vi "MAIN_All_In_One.vi"() -> ()   [LabVIEW 2019]
uses:
  States/Assessment_Modes.ctl
  States/Main_States.ctl
  States/Hand.ctl
  States/ROM_States.ctl
  <vilib>/myRIO/Common/Instrument Driver Framework/myRIO v1.0/Encoder/typedefs/Encoder Signal Mode.ctl
  Shared VIs/Messages/NewPatientNotifierArgs.ctl
  Shared VIs/ModelSpecific/ETHMikeModel.ctl
  Shared VIs/ModelSpecific/ReadOnlyGlobalActions.ctl
  <vilib>/myRIO/Instrument Drivers/Onboard IO/AI/typedefs/AI Reference.ctl
  <vilib>/myRIO/Common/Instrument Driver Framework/Utilities/typedefs/myRIO Generic Hardware Reference.ctl
  <vilib>/myRIO/Common/Instrument Driver Framework/Utilities/typedefs/Hardware Version Enum.ctl
  <vilib>/myRIO/Common/Instrument Driver Framework/Utilities/typedefs/myRIO v1.0 Reference.ctl
  <vilib>/myRIO/Common/Instrument Driver Framework/Utilities/typedefs/Generic FPGA Reference.ctl
  <vilib>/myRIO/Common/Instrument Driver Framework/myRIO v1.0/AI/typedefs/AI Channels List.ctl
  <vilib>/myRIO/Common/Instrument Driver Framework/myRIO v1.0/AI/typedefs/AI Channels Enum.ctl
  <vilib>/myRIO/Common/Instrument Driver Framework/Utilities/typedefs/Analog Scaling Constants List.ctl
  <vilib>/myRIO/Common/Instrument Driver Framework/Utilities/typedefs/Analog Scaling Constants.ctl
  <vilib>/userDefined/High Color/nirio_resource_hc.ctl
  <vilib>/myRIO/Instrument Drivers/Onboard IO/AO/typedefs/AO Reference.ctl
  <vilib>/myRIO/Common/Instrument Driver Framework/myRIO v1.0/AO/typedefs/AO Channels List.ctl
  <vilib>/myRIO/Common/Instrument Driver Framework/myRIO v1.0/AO/typedefs/AO Channels Enum.ctl
  <vilib>/Platform/TimedLoop/XDataNode/timing_clust.ctl
  <vilib>/Platform/TimedLoop/XDataNode/nitl_modes.ctl
  <vilib>/Platform/TimedLoop/XDataNode/wakeup.ctl
  Shared VIs/TypeDef_TDMS_States.ctl
  <vilib>/Analysis/3filter.llb/Filter Passband Type.ctl
  Shared VIs/Messages/UdpGlobalActions.ctl
  Shared VIs/ENPID/OutputRange.ctl
  Shared VIs/Messages/MsgHeader.ctl
  Shared VIs/Messages/PatientSelectMsg.ctl
  Shared VIs/Messages/CommandMsg.ctl
  Shared VIs/Messages/BackendInfoMsg.ctl
  <vilib>/myRIO/Common/Instrument Driver Framework/myRIO v1.0/AI/vis/myRIO v1.1 Open AI.vi
  <vilib>/myRIO/Common/Instrument Driver Framework/myRIO v1.0/AO/vis/myRIO v1.1 Open AO.vi
  <vilib>/myRIO/Common/Instrument Driver Framework/Utilities/vis/Validate Channels.vi
  <vilib>/myRIO/Common/Instrument Driver Framework/myRIO v1.0/AI/vis/myRIO v1.0 Reserve AI.vi
  <vilib>/myRIO/Common/Instrument Driver Framework/myRIO v1.0/AO/vis/myRIO v1.0 Reserve AO.vi
  <vilib>/myRIO/Common/Instrument Driver Framework/myRIO v1.0/AI/vis/myRIO v1.0 Close AI.vi
  <vilib>/myRIO/Common/Instrument Driver Framework/myRIO v1.0/AO/vis/myRIO v1.0 Close AO.vi
  <vilib>/myRIO/Common/Instrument Driver Framework/myRIO v1.0/Encoder/vis/myRIO v1.0 Close Encoder.vi
  <vilib>/myRIO/Common/Instrument Driver Framework/myRIO v1.0/AI/vis/myRIO v1.0 Build MUX Configuration AI.vi
  <vilib>/myRIO/Common/Instrument Driver Framework/myRIO v1.0/Resource Manager/vis/myRIO v1.0 Reserve Channel List.vi
  <vilib>/myRIO/Common/Instrument Driver Framework/myRIO v1.0/AO/vis/myRIO v1.0 Build MUX Configuration AO.vi
  <vilib>/myRIO/Common/Instrument Driver Framework/myRIO v1.0/AI/vis/myRIO v1.0 Unreserve AI.vi
  <vilib>/myRIO/Common/Instrument Driver Framework/myRIO v1.0/AO/vis/myRIO v1.0 Unreserve AO.vi
  <vilib>/myRIO/Common/Instrument Driver Framework/myRIO v1.0/Encoder/vis/myRIO v1.0 Unreserve Encoder.vi
  <vilib>/myRIO/Common/Instrument Driver Framework/myRIO v1.0/Resource Manager/vis/myRIO v1.0 Reserve Channel.vi
  <vilib>/myRIO/Common/Instrument Driver Framework/myRIO v1.0/Resource Manager/vis/myRIO v1.0 Unreserve Channel.vi
  <vilib>/myRIO/Common/Instrument Driver Framework/myRIO v1.0/Resource Manager/vis/myRIO v1.0 Unreserve Channel List.vi
  <vilib>/myRIO/Common/Instrument Driver Framework/myRIO v1.0/Encoder/vis/myRIO v1.0 Build MUX Configuration Encoder.vi
  <vilib>/myRIO/Common/Instrument Driver Framework/myRIO v1.0/Resource Manager/vis/myRIO v1.0 Build Mutex Name.vi
  <vilib>/myRIO/Common/Instrument Driver Framework/myRIO v1.0/Resource Manager/vis/myRIO v1.0 Create Configuration List.vi
  <vilib>/Utility/VariantDataType/GetNumericInfo.vi
  <vilib>/Utility/error.llb/Error Cluster From Error Code.vi
  <vilib>/myRIO/Common/Instrument Driver Framework/myRIO v1.0/myRIO v1.1 Open.vi
  <vilib>/myRIO/Common/Instrument Driver Framework/myRIO v1.0/AO/vis/myRIO v1.0 Get Scaling Constants AO.vi
  <vilib>/myRIO/Common/Instrument Driver Framework/Utilities/vis/IO Manager.vi
  <vilib>/myRIO/Common/Instrument Driver Framework/Utilities/vis/Configuration Manager.vi
  <vilib>/myRIO/Common/Instrument Driver Framework/myRIO v1.0/myRIO v1.0 Close.vi
  <vilib>/myRIO/Common/Instrument Driver Framework/myRIO v1.0/AO/vis/myRIO v1.0 Write AO.vi
  <vilib>/myRIO/Common/Instrument Driver Framework/myRIO v1.0/AI/vis/myRIO v1.0 Get Scaling Constants AI.vi
  <vilib>/myRIO/Common/Instrument Driver Framework/myRIO v1.0/AI/vis/myRIO v1.0 Read AI.vi
  <vilib>/myRIO/Common/Instrument Driver Framework/myRIO v1.0/Encoder/vis/myRIO v1.0 Read Encoder.vi
  <vilib>/functionblocks/Counter/Elapsed Timer/Elapsed Timer.vi
  <vilib>/myRIO/Common/Instrument Driver Framework/myRIO v1.0/Encoder/vis/myRIO v1.0 Enable Encoder.vi
  <vilib>/myRIO/Common/Instrument Driver Framework/myRIO v1.0/Encoder/vis/myRIO v1.0 Shutdown Encoder.vi
  <vilib>/myRIO/Common/Instrument Driver Framework/myRIO v1.0/Resource Manager/vis/myRIO v1.0 Configure IO.vi
  <vilib>/myRIO/Instrument Drivers/Onboard IO/AO/vis/myRIO AO Open.xnode
  <vilib>/myRIO/Instrument Drivers/Onboard IO/AI/vis/myRIO AI Open.xnode
  <vilib>/platform/TimedLoop/XDataNode/XDataNode.xnode
  <vilib>/functionblocks/FB Core/FB Core.xnode
  <vilib>/myRIO/Instrument Drivers/Onboard IO/AO/AO.lvlib
  <vilib>/myRIO/Instrument Drivers/Onboard IO/Encoder/Encoder.lvlib
  <vilib>/myRIO/Instrument Drivers/Onboard IO/AI/AI.lvlib
  <vilib>/Platform/TimedLoop/XDataNode/XDNodeRunTimeDep.lvlib
  <vilib>/functionblocks/NI_FunctionBlock Libraries.lvlib
  <vilib>/addons/control/pid/NI_PID_pid.lvlib
  <vilib>/Analysis/NI_AALBase.lvlib
  <vilib>/ptbypt/NI_PtbyPt.lvlib
panel:
  out "SkipSignal":bool
  out "Force_calib_value":dbl
  out "Velocity_calib_value":dbl
  out "LogFileOpen":bool
  out "Phase Trial Count":i16
  out "Error which lead\nto TCP close":errorcluster
  out "TCP Error":errorcluster
  out "UDP Error":errorcluster
  in  "stop":bool
  out "SelectedHand":T1
  out "Connected":bool
  out "Remote IP":u32 format="%x"
  out "StopRequested":bool
  in  "TCP Server Port":u16=6662
  in  "UDP Destination Port":u16=6661
  out "DateTime":string
  out "SubjectNr":string
  out "StopSignal":bool
  out "RestartSignal":bool
  out "StartSignal":bool
  out "FrontendStartedSignal":bool
  out "Flexion":bool
  out "AssessmentFinished":bool
  out "ROM State":T2=enum."Passive"
  out "LeftHand":bool
  out "Task State":T3=enum."Start"
  out "MovingToTarget":bool=TRUE
  out "ROM max":dbl
  out "ROM min":dbl
  out "Zero Position":dbl
  out "Largest USB Partition Path":path
  out "Velocity unfiltered [deg/s]":dbl
  out "Trial Nr":i16
  out "Starting position":dbl
  out "Target Array":dbl[](array[numeric])
  out "AssessmentMode":T4
  out "Current Setpoint [A]":dbl
  out "Finished late?":bool
  out "Position [deg]":dbl
  out "Velocity [deg/s]":dbl
  out "Current [A]":dbl
  out "Time (s)":dbl
  out "Voltage force":dbl
  out "Force":dbl
  out "Force filtered":dbl
  out "Target state?":bool
  out "Target Position [deg]":dbl
  # "Frontend Connection"
  # "Command Signals"
  # "Motor State"
  # "Patient Data"
  # "Assessment State"
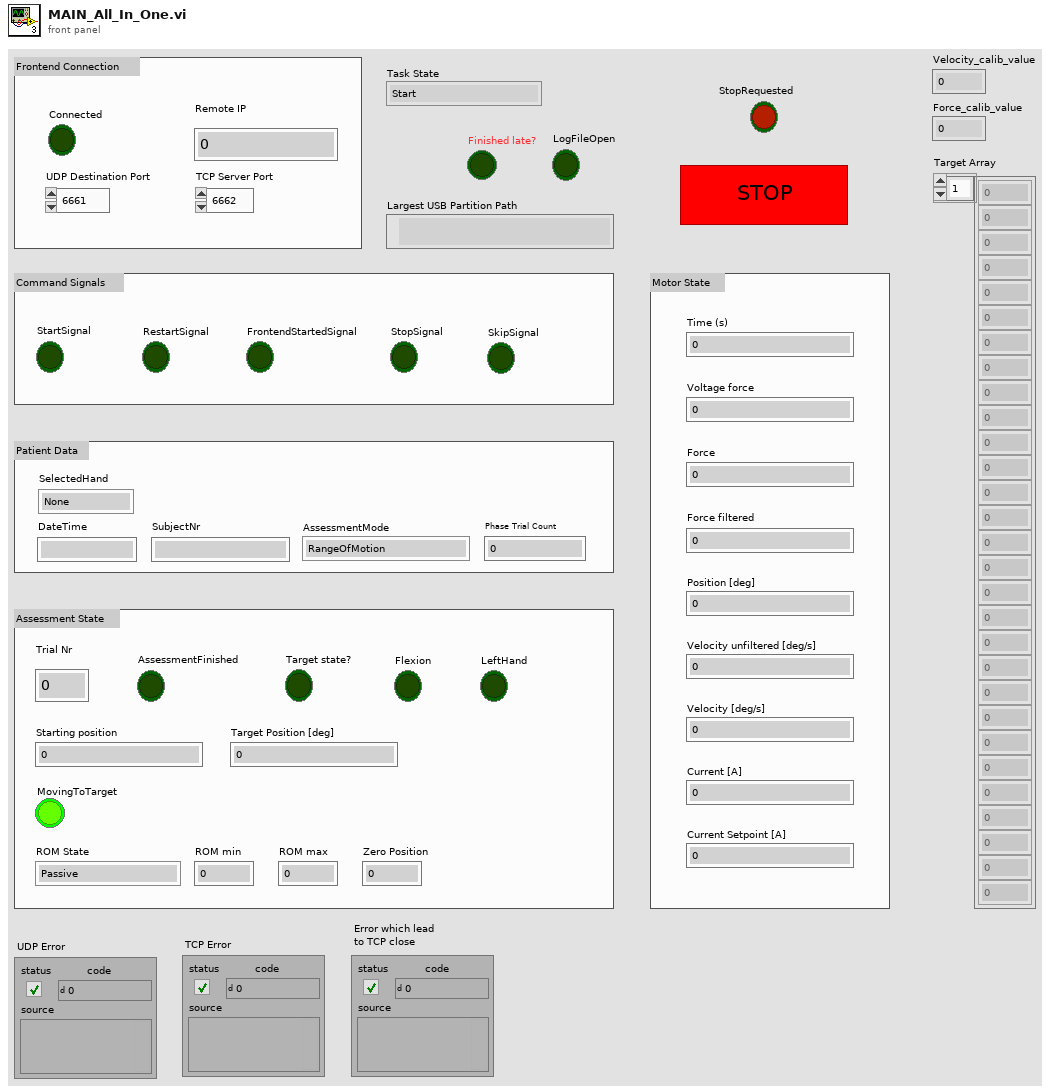
[diagram p1: front panel]
types:
  T1 = typedef "Hand.ctl" = enum8{"None", "Left", "Right"}
  T2 = typedef "ROM_States.ctl" = enum8{"Active", "Passive", "AutomaticPassive"}
  T3 = typedef "Main_States.ctl" = enum16{"Hand choice", "Start", "Show target", "Resetting", "WaitingForRestart"}
  T4 = typedef "Assessment_Modes.ctl" = enum8{"RangeOfMotion", "Force", "Motor", "Sensorimotor", "PositionMatching", "PreciseReaching"}
  T5 = typedef "NewPatientNotifierArgs.ctl" = cluster{"Left":bool, "Mode":T4, "Name":string, "Timestamp":string, "StudyName":string}
  T6 = cluster{"read mode":enum16{"polling", "blocking"}, "write mode":enum16{"polling", "blocking"}}
  T7 = typedef "nirio_resource_hc.ctl" = tag
  T8 = typedef "Hardware Version Enum.ctl" = enum16{"Unknown", "myRIO-1900", "myRIO-1950", "roboRIO", "NI ELVIS RIO CM", "ELVIS III"}
  T9 = typedef "TypeDef_TDMS_States.ctl" = enum16{"WaitingForCreate", "Create", "Buffering", "Flushing", "Write", "Close"}
  T10 = enum16{"open", "open or create", "create or replace", "create", "open (read-only)"}
  T11 = typedef "XDNodeRunTimeDep.lvlib/timing_clust.ctl" = cluster{"Expected End [f-1]":u64, "Actual End [f-1]":u64, "Finished Late? [f-1]":bool, "Expected End [i-1]":u64, "Actual End [i-1]":u64, "Finished Late? [i-1]":bool, "Expected Start [i]":u64, "Actual Start [i]":u64, "Expected Start [f]":u64, "Actual Start [f]":u64, "Source Name":string, "Structure Name":string, "Period":i64, "Deadline":i64, "Offset":i64, "Start":i64, "Priority":i32, "Timeout":i32, "Mode":T12, "Wakeup Reason":T13, "Error":errorcluster, "Source Type":string, "Secondary Source Type":string, "Global End Time":u64, "Global Start Time":u64, "Frame Duration":u64, "Iteration Duration":u64, "Assigned CPU":i32, "I/O Scan Engine Mode":u32}
  T12 = typedef "XDNodeRunTimeDep.lvlib/nitl_modes.ctl" = enum32{"No Change", "Process missed periods, maintain original phase", "Discard missed periods, maintain original phase", "Process missed periods, ignore original phase", "Discard missed periods, ignore original phase"}
  T13 = typedef "XDNodeRunTimeDep.lvlib/wakeup.ctl" = enum32{"Normal", "Aborted", "Asynchronous wakeup", "Timing source error", "Timed loop error", "Timeout"}
  T14 = enum8{"Invalid", "PatientSelect", "Command", "Skip", "BackendInfoReq", "UnknownOp (Must be Last)"}
  T15 = typedef "MsgHeader.ctl" = cluster{"MsgType [0]":u8, "MsgLen [1:2]":u16}
  T16 = typedef "PatientSelectMsg.ctl" = cluster{"LeftHand":bool, "AssessmentMode":u8, "SubjectNr":string, "DateTime":string, "PhaseTrialCount":i32, "StudyName":string}
  T17 = typedef "CommandMsg.ctl" = cluster{"EmergencyStop":bool, "Start":bool, "Restart":bool, "FrontendStarted":bool, "Close":bool}
  T18 = typedef "BackendInfoMsg.ctl" = cluster{"ProtocolVersion":u16, "DataPath":string}
  T19 = typedef "UdpGlobalActions.ctl" = enum16{"Read", "Write"}
  T20 = typedef "NI_AALBase.lvlib/Filter Passband Type.ctl" = enum32{"Lowpass", "Highpass", "Bandpass", "Bandstop"}
  T21 = typedef "ReadOnlyGlobalActions.ctl" = enum16{"Initialize", "Read"}
  T22 = typedef "ETHMikeModel.ctl" = enum16{"ETH Mike #1", "ETH Mike #2", "ETH Mike #3", "ETH Mike #4", "ETH MIKE #5"}
  T23 = typedef "Encoder Signal Mode.ctl" = enum16{"Quadrature phase signal", "Step and direction signal"}
  T24 = typedef "AO.lvlib/AO Reference.ctl" = cluster{"myRIO Reference":T25, "AO Channel List":T28, "AO Scaling Constant List":T30}
  T25 = typedef "myRIO Generic Hardware Reference.ctl" = cluster{"myRIO Model":T8, "myRIO Hardware Reference":T26}
  T26 = typedef "myRIO v1.0 Reference.ctl" = cluster{"Generic FPGA Reference":T27, "Allow multiple opens":bool}
  T27 = typedef "Generic FPGA Reference.ctl" = refnum<k20>
  T28 = typedef "AO Channels List.ctl" = T29[]
  T29 = typedef "AO Channels Enum.ctl" = enum16{"Not Connected", "AudioOut/Left", "AudioOut/Right", "C/AO0", "C/AO1", "A/AO0", "A/AO1", "B/AO0", "B/AO1"}
  T30 = typedef "Analog Scaling Constants List.ctl" = T31[]
  T31 = typedef "Analog Scaling Constants.ctl" = cluster{"LSB Weight (Volts)":dbl, "Offset (Volts)":dbl, "Signed?":bool}
  T32 = typedef "Encoder.lvlib/Encoder Reference.ctl" = cluster{"myRIO Reference":T25, "Encoder Channels Enum":T33}
  T33 = typedef "Encoder Channels Enum.ctl" = enum16{"Not Connected", "C/ENC0", "C/ENC1", "A/ENC", "A/ENC0", "A/ENC1", "A/ENC2", "A/ENC3", "A/ENC4", "A/ENC5", "A/ENC6", "A/ENC7", "A/ENC8", "A/ENC9", "B/ENC", "B/ENC0", "B/ENC1", "B/ENC2", "B/ENC3", "B/ENC4", "B/ENC5", "B/ENC6", "B/ENC7", "B/ENC8", "B/ENC9", "DIO/ENC0", "DIO/ENC1", "DIO/ENC2", "DIO/ENC3", "DIO/ENC4"}
  T34 = typedef "AI.lvlib/AI Reference.ctl" = cluster{"myRIO Reference":T25, "AI Channels List":T35, "AI Scaling Constants List":T30}
  T35 = typedef "AI Channels List.ctl" = T36[]
  T36 = typedef "AI Channels Enum.ctl" = enum16{"Not Connected", "AudioIn/Left", "AudioIn/Right", "C/AI0", "C/AI1", "A/AI0", "A/AI1", "A/AI2", "A/AI3", "A/AI4", "A/AI5", "A/AI6", "A/AI7", "B/AI0", "B/AI1", "B/AI2", "B/AI3", "B/AI4", "B/AI5", "B/AI6", "B/AI7", "AI/AI0", "AI/AI1", "AI/AI2", "AI/AI3", "A/AI0 (DIFF)", "A/AI1 (DIFF)", "A/AI2 (DIFF)", "A/AI3 (DIFF)", "B/AI0 (DIFF)", "B/AI1 (DIFF)", "B/AI2 (DIFF)", "B/AI3 (DIFF)"}
  T37 = typedef "LVAllMonitorsDisplayTypeDef.ctl" = cluster{"Bounds":cluster{"Left":i16, "Top":i16, "Right":i16, "Bottom":i16}, "Depth":i16}[]
  T38 = cluster{"Bounds":cluster{"Left":i16, "Top":i16, "Right":i16, "Bottom":i16}, "Depth":i16}
  T39 = cluster{"Left":i16, "Top":i16, "Right":i16, "Bottom":i16}
  T40 = enum16{"Standard", "Buffered", "CRLF", "Immediate"}
  T41 = typedef "UDPRobotState.ctl" = cluster{"Counter":u32, "Time":sgl, "Position":sgl, "StartingPosition":sgl, "TargetPosition":sgl, "Force":sgl, "TrialNr":u8, "RomState":u8, "TargetState":bool, "Finished":bool, "Flexion":bool}
  T42 = typedef "OutputRange.ctl" = cluster{"output high":dbl, "output low":dbl}
  T43 = typedef "Gains.ctl" = cluster{"K(e)":dbl, "Kp":dbl, "Ki":dbl, "Kd":dbl}
  T44 = typedef "NonLinearGainParams.ctl" = cluster{"Non-linear gain P":T45, "Non-linear gain I":T45, "Non-linear gain D":T45}
  T45 = typedef "NonLinearGain.ctl" = enum16{"exponential", "quadratic", "off"}
  T46 = typedef "DPartVariable.ctl" = enum16{"error", "process variable"}
  T47 = typedef "VelocityEstimate.ctl" = enum16{"derivative", "external"}
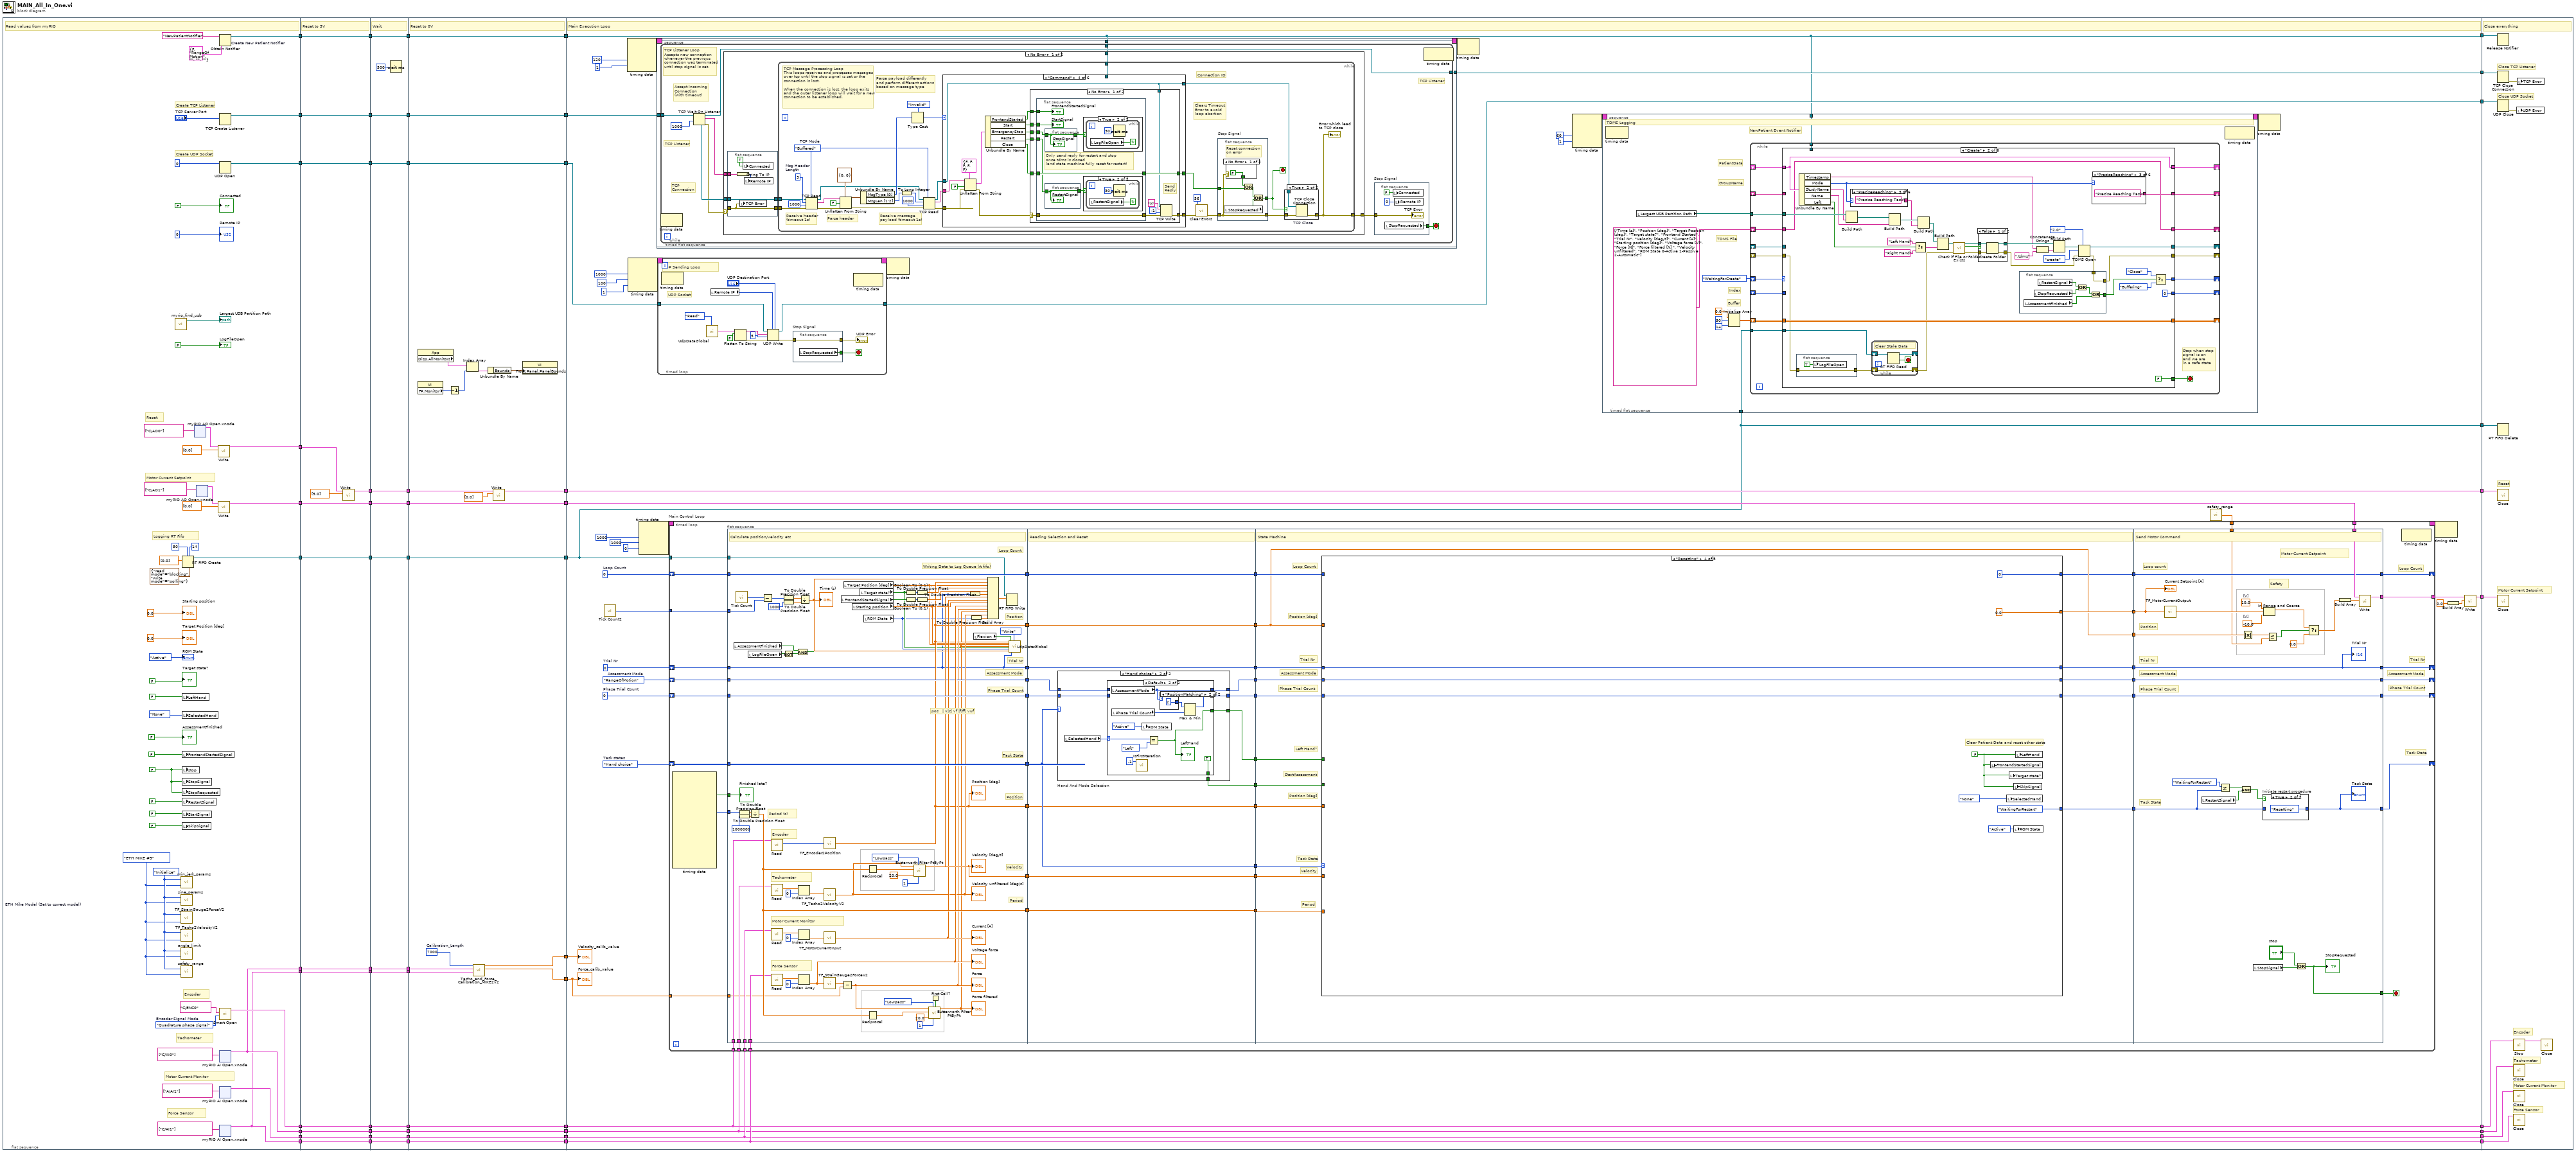
[diagram p0: block diagram]
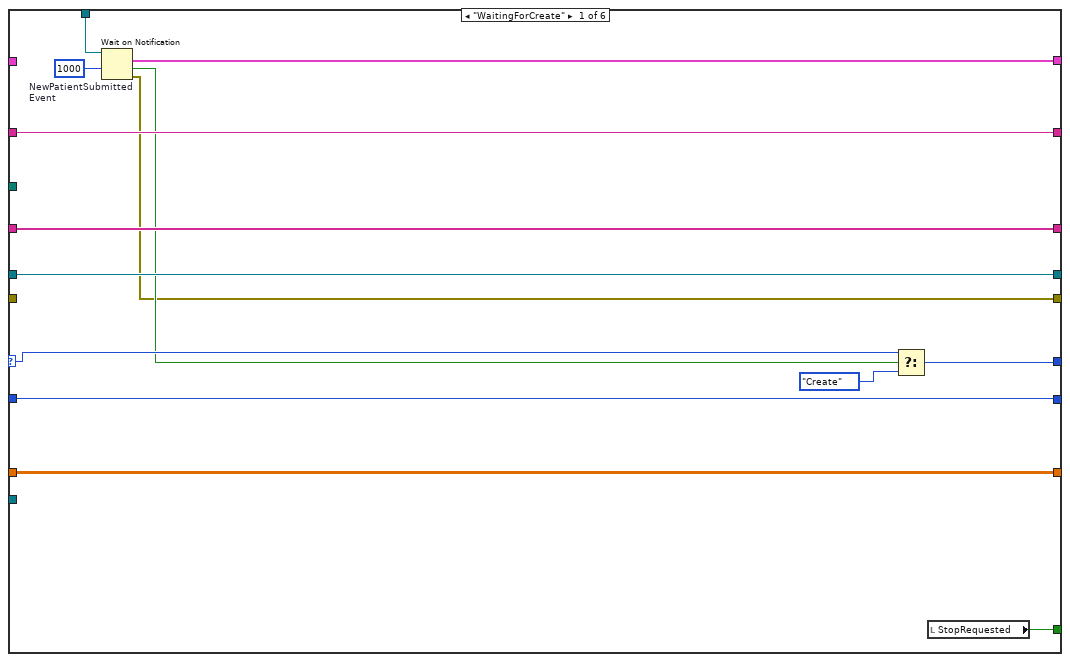
[diagram p2: hidden frame]
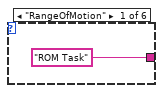
[diagram p3: hidden frame]
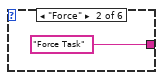
[diagram p4: hidden frame]
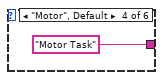
[diagram p5: hidden frame]
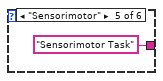
[diagram p6: hidden frame]
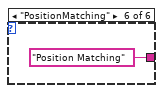
[diagram p7: hidden frame]
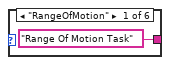
[diagram p9: hidden frame]
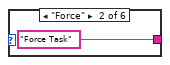
[diagram p10: hidden frame]
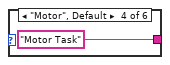
[diagram p11: hidden frame]
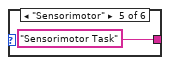
[diagram p12: hidden frame]
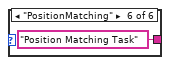
[diagram p13: hidden frame]
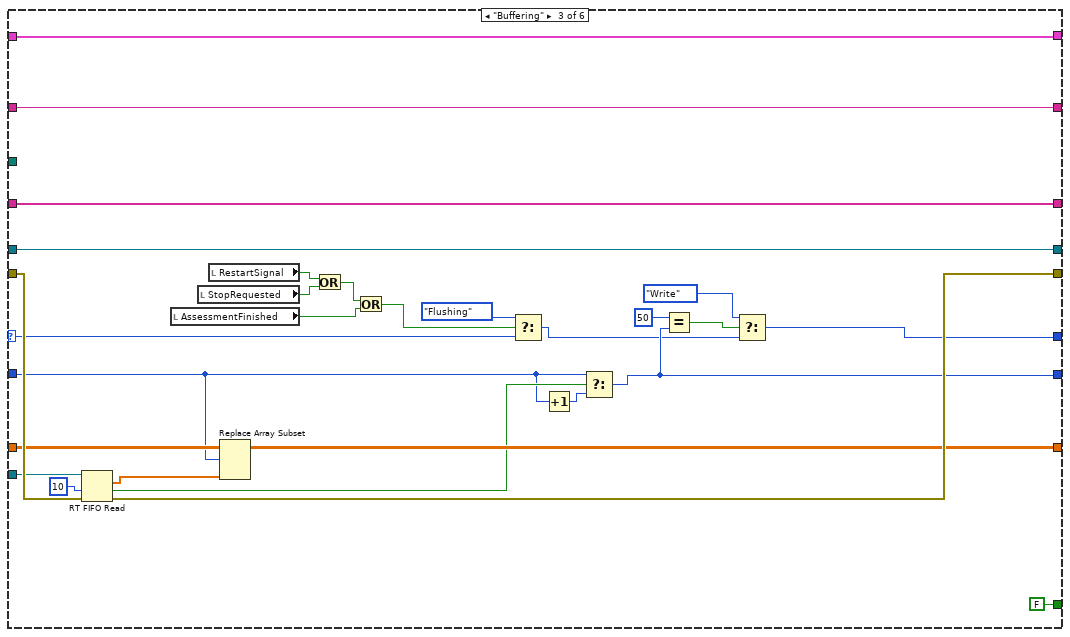
[diagram p14: hidden frame]
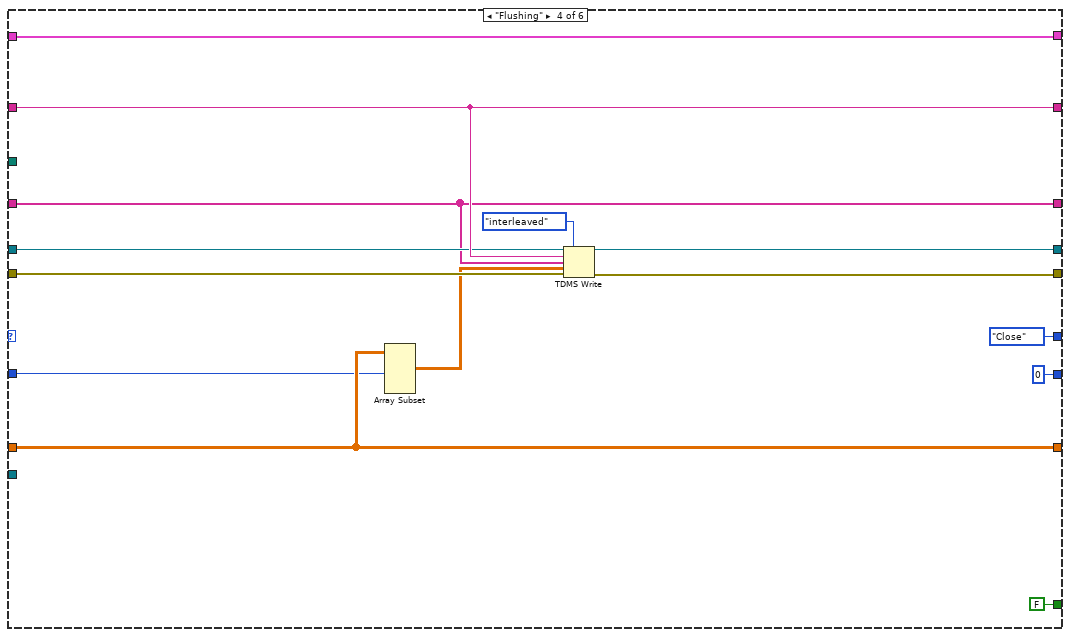
[diagram p15: hidden frame]
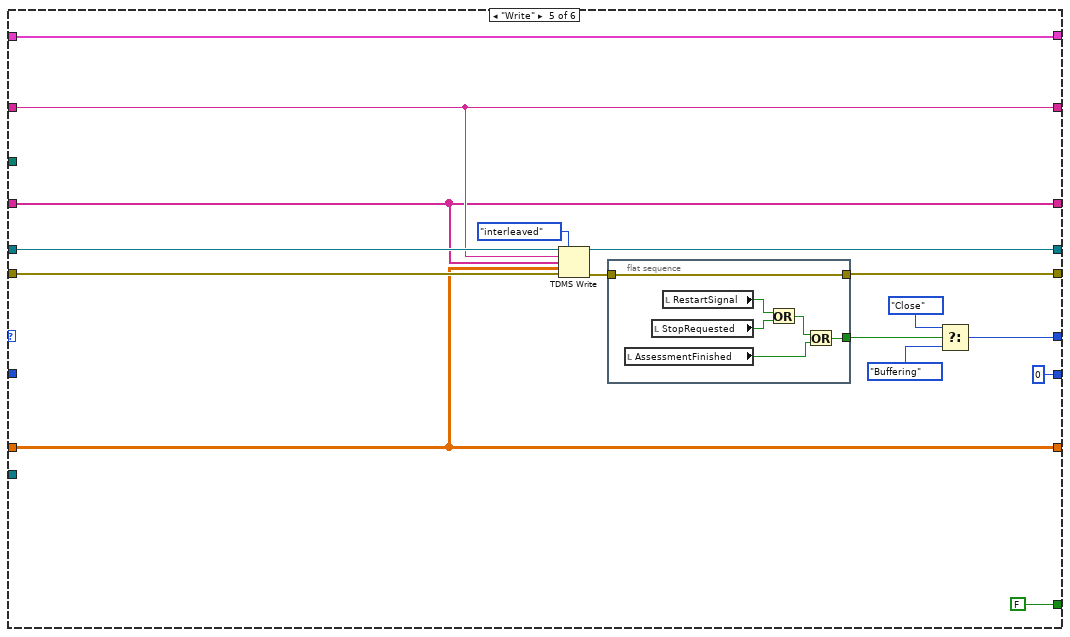
[diagram p16: hidden frame]
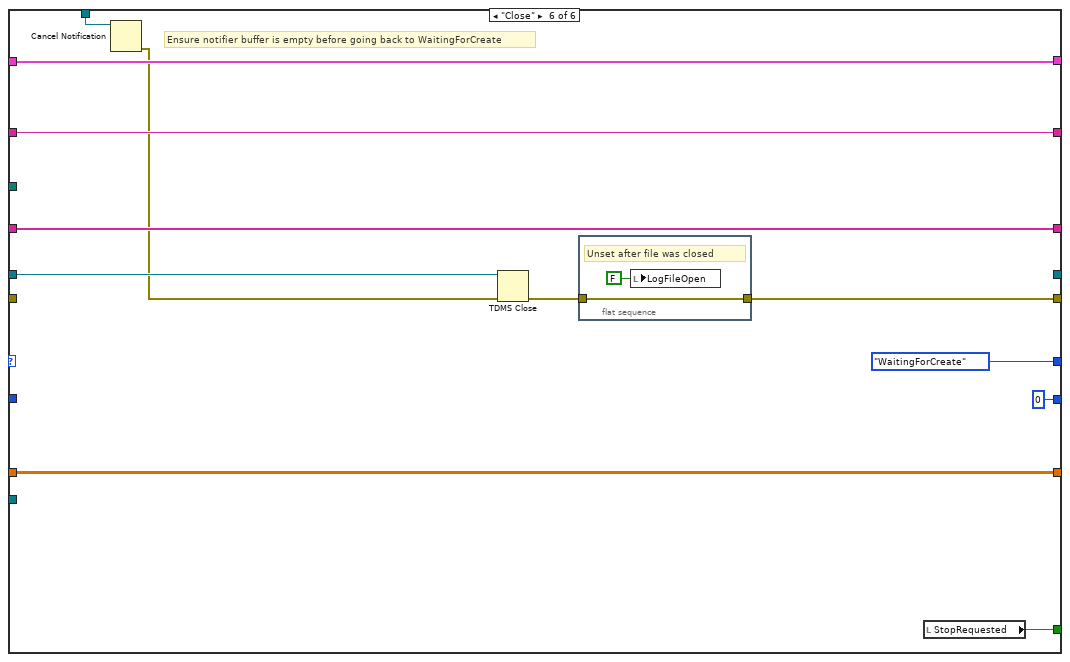
[diagram p17: hidden frame]
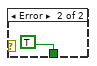
[diagram p19: hidden frame]
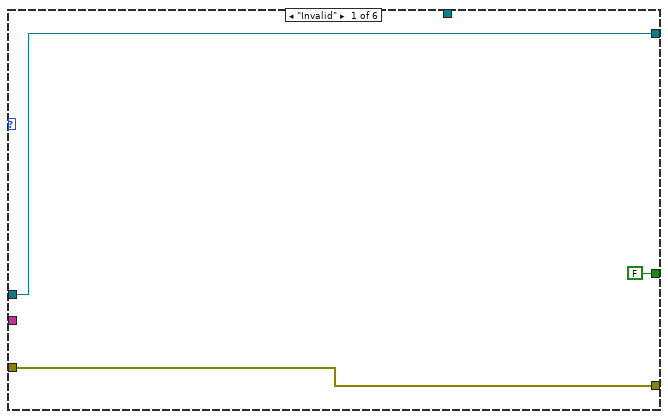
[diagram p20: hidden frame]
diagram:
  n1 = flat-sequence {
    tunnel: [w95] -> w58
    tunnel: [w94] -> w57
    tunnel: [w93] -> w56
    tunnel: [w92] -> w55
    tunnel: [w65] -> w54
    tunnel: [w64] -> w53
    tunnel: [w82] -> w25
    tunnel: [w80] -> w21
    tunnel: [w69] -> w15
    tunnel: [w68] -> w11
    tunnel: [w65] -> w6
    tunnel: [w64] -> w3
    tunnel: w58 -> [w208]
    tunnel: w57 -> [w206]
    tunnel: w56 -> [w205]
    tunnel: w55 -> [w204]
    tunnel: w54 -> [w203]
    tunnel: [w207] -> w52
    tunnel: [w206] -> w51
    tunnel: [w205] -> w50
    tunnel: [w204] -> w49
    tunnel: [w203] -> w48
    tunnel: [w202] -> w47
    tunnel: w53 -> [w202]
    tunnel: [w201] -> w26
    tunnel: w25 -> [w201]
    tunnel: [w200] -> w22
    tunnel: w21 -> [w200]
    tunnel: [w199] -> w16
    tunnel: w15 -> [w199]
    tunnel: [w198] -> w12
    tunnel: w11 -> [w198]
    tunnel: [w197] -> w7
    tunnel: w6 -> [w197]
    tunnel: [w196] -> w4
    tunnel: w3 -> [w196]
    tunnel: w52 -> [w217]
    tunnel: w51 -> [w222]
    tunnel: [w222] -> w46
    tunnel: [w221] -> w45
    tunnel: w50 -> [w221]
    tunnel: [w220] -> w44
    tunnel: w49 -> [w220]
    tunnel: [w219] -> w43
    tunnel: w48 -> [w219]
    tunnel: [w217] -> w42
    tunnel: [w216] -> w41
    tunnel: w47 -> [w216]
    tunnel: [w215] -> w27
    tunnel: w26 -> [w215]
    tunnel: [w214] -> w23
    tunnel: w22 -> [w214]
    tunnel: [w213] -> w17
    tunnel: w16 -> [w213]
    tunnel: [w212] -> w13
    tunnel: w12 -> [w212]
    tunnel: [w211] -> w8
    tunnel: w7 -> [w211]
    tunnel: [w210] -> w5
    tunnel: w4 -> [w210]
    tunnel: w46 -> [w241]
    tunnel: w45 -> [w240]
    tunnel: w44 -> [w239]
    tunnel: w43 -> [w238]
    tunnel: w42 -> [w243]
    tunnel: [w242] -> w40
    tunnel: [w241] -> w39
    tunnel: [w240] -> w38
    tunnel: [w239] -> w37
    tunnel: [w238] -> w36
    tunnel: [w237] -> w35
    tunnel: w41 -> [w237]
    tunnel: [w231] -> w28
    tunnel: w27 -> [w231]
    tunnel: w23 -> [w230]
    tunnel: [w230] -> w20
    tunnel: [w229] -> w18
    tunnel: w17 -> [w229]
    tunnel: [w228] -> w14
    tunnel: w13 -> [w228]
    tunnel: w8 -> [w227]
    tunnel: w5 -> [w225]
    tunnel: [w224] -> w2
    tunnel: [w223] -> w1
    tunnel: w40 -> [w284]
    tunnel: w39 -> [w254]
    tunnel: w38 -> [w285]
    tunnel: w37 -> [w252]
    tunnel: w36 -> [w251]
    tunnel: [w248] -> w34
    tunnel: [w254] -> w33
    tunnel: [w284] -> w32
    tunnel: [w251] -> w31
    tunnel: [w252] -> w30
    tunnel: w35 -> [w253]
    tunnel: [w253] -> w29
    tunnel: w28 -> [w276]
    tunnel: [w264] -> w24
    tunnel: w20 -> [w275]
    tunnel: [w263] -> w19
    tunnel: w18 -> [w261]
    tunnel: w14 -> [w256]
    tunnel: [w256] -> w10
    tunnel: [w261] -> w9
    tunnel: w2 -> [w255]
    tunnel: w1 -> [w245]
    tunnel: w34 -> [w1505]
    tunnel: w33 -> [w1516]
    tunnel: w32 -> [w1515]
    tunnel: w31 -> [w1512]
    tunnel: w30 -> [w1514]
    tunnel: w29 -> [w1513]
    tunnel: w24 -> [w1511]
    tunnel: w19 -> [w1510]
    tunnel: w10 -> [w1507]
    tunnel: w9 -> [w1506]
    frame #0 {
      w60 = ReadOnlyGlobalActions."Initialize" ("Action (Read)")
      w59 = ETHMikeModel."ETH MIKE #5"  # ETH Mike Model (Set to correct model)
      w76 = FALSE ("stop")
      w101 = Encoder_Signal_Mode."Quadrature phase signal"  # Encoder Signal Mode
      # "Logging RT Fifo"
      # "Create TCP Listener"
      # "Create UDP Socket"
      # "Force Sensor"
      # "Tachometer"
      # "Motor Current Monitor"
      # "Motor Current Setpoint"
      # "Reset"
      # "Encoder"
      # "Read values from myRIO"
      n2 = call "myrio_find_usb.vi"() -> ("Largest USB Partition Path"=→"Largest USB Partition Path":path)  [unwired: 9 in, 2 out]
      n3 = call "min_jerk_params.vi"("Action (Read)"=w60, "ETH Mike Model"=w59) -> ()  [unwired: 12 in, 6 out]
      n4 = call "sine_params.vi"("Action (Read)"=w60, "ETH Mike Model"=w59) -> ()  [unwired: 12 in, 6 out]
      n5 = call "TF_StrainGauge2ForceV2.vi"("Action (Read)"=w60, "ETH Mike Model"=w59) -> ()  [unwired: 3 in, 1 out]
      n6 = call "TF_Tacho2VelocityV2.vi"("Action (Read)"=w60, "ETH Mike Model"=w59) -> ()  [unwired: 3 in, 1 out]
      n7 = call "angle_limit.vi"("ETH Mike Model"=w59, "Action (Read)"=w60) -> ()  [unwired: 1 out]
      n8 = call "safety_range.vi"("ETH Mike Model"=w59, "Action (Read)"=w60) -> ()  [unwired: 1 out]
      n9 = RT FIFO Create(1:dbl[] [0.0] ("Values"), 4:u32 50 ("size (10)"), 6:u32 14 ("elements in array (1)"), 7:T6 {"read mode"=enum."blocking", "write mode"=enum."polling"} ("r/w modes (polling,polling)")) -> (8:w69:refnum<k33>)  [unwired: 4 in, 2 out]
      n10 = local write "LeftHand"(FALSE ("Right")) -> ()
      n11 = local write "SelectedHand"(Hand."None" ("Enum")) -> ()
      n12 = local write "FrontendStartedSignal"(FALSE) -> ()
      n13 = local write "stop"(w76) -> ()
      n14 = local write "StopSignal"(w76) -> ()
      n15 = local write "StopRequested"(w76) -> ()
      n16 = local write "RestartSignal"(FALSE ("Restart")) -> ()
      n17 = local write "StartSignal"(FALSE ("StartSignal")) -> ()
      n18 = local write "SkipSignal"(FALSE ("StartSignal")) -> ()
      n19 = xnode "myRIO AO Open.xnode"("Channel Names"=tag[] ["C/AO0"]) -> ("AO Ref Out"=w104:T24)  [unwired: 2 in, 1 out]
      n20 = xnode "myRIO AO Open.xnode"("Channel Names"=tag[] ["C/AO1"]) -> ("AO Ref Out"=w99:T24)  [unwired: 2 in, 1 out]
      n21 = call <vilib>:"Write.vi"("Values"=dbl[] [0.0], "AO Ref In"=w104) -> ("AO Ref Out"=w95:T24)  [unwired: 7 in, 1 out]
      n22 = call <vilib>:"Write.vi"("Values"=dbl[] [0.0], "AO Ref In"=w99) -> ("AO Ref Out"=w93:T24)  [unwired: 7 in, 1 out]
      n23 = Obtain Notifier "Create New Patient Notifier"(name (unnamed)="NewPatientNotifier", notification data type=T5 {"Left"=FALSE, "Mode"=enum."RangeOfMotion", "Name"="", "Timestamp"="", "StudyName"=""}) -> (notifier out=w68:refnum<notifier>)  [unwired: 2 in, 2 out]
      n24 = TCP Create Listener(10:"TCP Server Port") -> (3:w80:refnum<k5>)  [unwired: 4 in, 2 out]
      n25 = UDP Open(11:u16 0) -> (port=w82:refnum<k16>)  [unwired: 4 in, 2 out]
      n26 = call <vilib>:"Smart Open.vi"("Encoder Signal Mode"=w101, "Channel Name"=tag "C/ENC0") -> ("Encoder Ref Out"=w94:T32)  [unwired: 8 in, 1 out]
      n27 = xnode "myRIO AI Open.xnode"("Channel Names"=tag[] ["C/AI0"]) -> ("AI Ref Out"=w65:T34)  [unwired: 2 in, 1 out]
      n28 = xnode "myRIO AI Open.xnode"("Channel Names"=tag[] ["A/AI1"]) -> ("AI Ref Out"=w92:T34)  [unwired: 2 in, 1 out]
      n29 = xnode "myRIO AI Open.xnode"("Channel Names"=tag[] ["C/AI1"]) -> ("AI Ref Out"=w64:T34)  [unwired: 2 in, 1 out]
      "Target state?" <- FALSE ("Target state?")
      "Target Position [deg]" <- 0.0 ("Target Position [deg]")
      "ROM State" <- ROM_States."Active" ("Enum")
      "Connected" <- FALSE
      "Remote IP" <- u32 0
      "LogFileOpen" <- FALSE ("LogFileOpen")
      "AssessmentFinished" <- FALSE ("AssessmentFinished")
      "Starting position" <- 0.0 ("Starting position")
    }
    frame #1 {
      # "Reset to 5V"
      n30 = call <vilib>:"Write.vi"("Values"=dbl[] [5.0], "AO Ref In"=w208) -> ("AO Ref Out"=w207:T24)  [unwired: 7 in, 1 out]
    }
    frame #2 {
      # "Wait"
      n31 = Wait (ms)(milliseconds to wait=u32 500) -> ()  [unwired: 1 out]
    }
    frame #3 {
      w226 = 7000  # Calibration_Length
      # "Reset to 0V"
      n32 = property class="App"() -> ("Disp.AllMonitors"=w236:T37)  [unwired: 2 in, 2 out]
      n33 = property class="VI"() -> ("FP.Monitor"=w235:u16)  [unwired: 2 in, 2 out]
      n34 = Decrement(x=w235) -> (x-1=w234:u16)
      n35 = Index Array(array=w236, index=w234) -> (element=w233:T38)
      n36 = call "Tacho_and_Force_Calibration_MIKE2v2.vi"("Force Ref In"=w225, "Tacho Ref In"=w227, "Calibration_Length"=w226) -> ("Force_calib_value"=w223:dbl, "Velocity_calib_value"=w224:dbl)  [unwired: 7 in]
      n37 = Unbundle By Name(w233) -> ("Bounds"=w232:T39)
      n38 = call <vilib>:"Write.vi"("Values"=dbl[] [0.0], "AO Ref In"=w243) -> ("AO Ref Out"=w242:T24)  [unwired: 7 in, 1 out]
      n39 = property class="VI"("Front Panel.PanelBounds"=w232) -> ()  [unwired: 2 in, 2 out]
    }
    frame #4 {
      w265 = Assessment_Modes."RangeOfMotion"  # Assessment Mode
      w266 = i16 0  # Phase Trial Count
      w279 = i16 0  # Trial Nr
      w280 = Main_States."Hand choice"  # Task states
      w262 = 0  # Loop Count
      # "Main Execution Loop"
      n40 = call "Tick Count2"() -> ("Tick Count(mSec)"=w282:u32)
      n41 = node-c288(120 ("Priority"), 1 ("Processor")) -> (w272:T11)  [unwired: 2 in]
      n42 = node-c288(i64 1000 ("Period"), 100 ("Priority"), 1 ("Processor")) -> (w278:T11)  [unwired: 1 in]
      n43 = node-c288(i64 1000 ("Period"), 1000 ("Priority"), 0 ("Processor")) -> (w287:T11)  [unwired: 1 in]
      n44 = timed-sequence {
        timing: w272 -> [_]
        timing-out: [_] -> w271
        tunnel: w275 -> [w490]
        tunnel: [w489] -> w263
        tunnel: w256 -> [w488]
        n45 = timed-flat-sequence {
          tunnel: w490 -> [w493]
          tunnel: [w492] -> w489
          tunnel: w488 -> [w491]
          n46 = node-c288() -> ()  [unwired: 1 in, 1 out]
          n47 = while {
            tunnel: w493 -> [w504]
            tunnel: [w497] -> w492
            tunnel: w491 -> [w496]
            stop <- w499 stop-if-true
            # "TCP Listener"
            # "TCP Listener"
            # "TCP \nConnection"
            # "TCP Listener Loop\nAccepts new connection\nwhenever the previous\nconnection was terminated\nuntil stop signal is set."
            # "Accept Incoming\nConnection\n(with timeout)"
            n48 = TCP Wait On Listener ("TCP Accept")(9:1000, 11:w504) -> (0:w502:errorcluster, 2:w498:string, 3:w497:refnum<k5>, 4:w503:refnum<k5>)  [unwired: 2 in, 1 out]
            n49 = case shown="No Error" w502 {
              selector: w502 -> [w514 w690]
              tunnel: w503 -> [w512 _]
              tunnel: [w515 w690] -> w500
              tunnel: w498 -> [w510 _]
              tunnel: w496 -> [w509 _]
              frame No Error {
                n50 = flat-sequence {
                  tunnel: w514 -> [w516]
                  tunnel: [w516] -> w513
                  tunnel: w512 -> [w518]
                  tunnel: [w518] -> w511
                  tunnel: w510 -> [w517]
                  frame #0 {
                    n51 = String To IP(1:w517) -> (0:w520:u32)
                    n52 = local write "TCP Error"(w516) -> ()
                    n53 = local write "Connected"(TRUE) -> ()
                    n54 = local write "Remote IP"(w520) -> ()
                  }
                }
                n55 = while {
                  tunnel: w513 -> [w541]
                  tunnel: w511 -> [w540]
                  tunnel: [w526] -> w515
                  tunnel: w509 -> [w521]
                  stop <- w533 stop-if-true
                  w527 = T40."Buffered"  # TCP Mode
                  w547 = 3  # Msg Header Length
                  # "Connection ID"
                  # "Clears Timeout \nError to avoid \nloop abortion"
                  # "TCP Message Processing Loop\nThis loops receives and processes messages\nover tcp until the stop signal is set or the\nconnection is lost.\n\nWhen the connection is lost, the loop exits\nand the outer listener loop will wait for a new\nconnection to be established."
                  # "Parse payload differently\nand perform different actions\nbased on message type"
                  # "Parse header"
                  # "Receive message \npayload (timeout 1s)"
                  # "Receive header\n(timeout 1s)"
                  n56 = TCP Read(connection ID=w540, bytes to read=w547, error in (no error)=w541, 7:w527, 9:1000) -> (connection ID out=w535:refnum<k5>, data out=w549:string, error out=w546:errorcluster)
                  n57 = Unflatten From String(type=T15 {"MsgType [0]"=0, "MsgLen [1:2]"=0} ("Msg Header \nFormat"), binary string=w549, data includes array or string size? (T)=FALSE, error in (no error)=w546) -> (value=w545:T15, error out=w539:errorcluster)  [unwired: 1 in, 1 out]
                  n58 = Unbundle By Name(w545) -> ("MsgType [0]"=w543:u8, "MsgLen [1:2]"=w531:u16)
                  n59 = To Long Integer(number=w531) -> (32bit integer=w538:i32)
                  n60 = Type Cast(type=T14."Invalid", x=w543) -> (*(type *) &x=w537:T14)
                  n61 = TCP Read(connection ID=w535, bytes to read=w538, error in (no error)=w539, 7:w527, 9:1000) -> (connection ID out=w523:refnum<k5>, data out=w536:string, error out=w529:errorcluster)
                  n62 = case shown="\"Command\"" w537 {
                    tunnel: w529 -> [w564 w570 w586 w633 w667 w686]
                    tunnel: w536 -> [_ _ w587 w634 _ _]
                    tunnel: [FALSE ("Close") FALSE ("Close") FALSE w630 FALSE ("Close") FALSE ("Close")] -> w534
                    tunnel: [w564 w569 w578 w624 w669 w688] -> w524
                    tunnel: w523 -> [w563 w567 w577 w625 w666 w684]
                    tunnel: [w563 w566 w577 w625 w666 w683] -> w522
                    tunnel: w521 -> [_ _ w575 _ _ _]
                    frame "Invalid" {
                    }
                    frame Default {
                      # "In case of an unknown message type,\nsend '?' as reply, so the frontend can detect the version incompatibility and display an error."
                      # "Send\nReply"
                      n63 = TCP Write(connection ID=w567, data in="?", error in (no error)=w570, 9:-1 ("timeout ms (25000)")) -> (connection ID out=w566:refnum<k5>, error out=w569:errorcluster)  [unwired: 1 out]
                    }
                    frame "PatientSelect" {
                      n64 = Unflatten From String(type=T16 {"LeftHand"=FALSE, "AssessmentMode"=0, "SubjectNr"="", "DateTime"="", "PhaseTrialCount"=0, "StudyName"=""}, binary string=w587, data includes array or string size? (T)=FALSE, error in (no error)=w586) -> (value=w584:T16, error out=w579:errorcluster)  [unwired: 1 in, 1 out]
                      n65 = Unbundle By Name(w584) -> ("LeftHand"=w583:bool, "AssessmentMode"=w582:u8, "SubjectNr"=w581:string, "DateTime"=w580:string, "PhaseTrialCount"=w576:i32, "StudyName"=w573:string)
                      n66 = case shown="No Error" w579 {
                        selector: w579 -> [w600 w623]
                        tunnel: w583 -> [w604 _]
                        tunnel: w582 -> [w603 _]
                        tunnel: w581 -> [w601 _]
                        tunnel: w580 -> [w602 _]
                        tunnel: [w599 w623] -> w578
                        tunnel: w577 -> [w596 _]
                        tunnel: w576 -> [w595 _]
                        tunnel: w575 -> [w591 _]
                        tunnel: w573 -> [w589 _]
                        frame No Error {
                          # "Send\nReply"
                          n67 = flat-sequence {
                            tunnel: w604 -> [w612]
                            tunnel: w603 -> [w611]
                            tunnel: w602 -> [w609]
                            tunnel: w601 -> [w610]
                            tunnel: w600 -> [w615]
                            tunnel: w595 -> [w605]
                            tunnel: [w615] -> w594
                            tunnel: [w614] -> w593
                            tunnel: [w608] -> w592
                            tunnel: w589 -> [w607]
                            tunnel: [w618] -> w598
                            tunnel: w594 -> [w619]
                            tunnel: w593 -> [w620]
                            tunnel: w592 -> [w622]
                            tunnel: w591 -> [w621]
                            frame #0 {
                              n68 = To Word Integer(number=w605) -> (16bit integer=→"Phase Trial Count":i16)
                              n69 = Bundle By Name(cluster=T5 {"Left"=FALSE, "Mode"=enum."RangeOfMotion", "Name"="", "Timestamp"="", "StudyName"=""}, "Left"=w612, "Mode"=w611, "Name"=w610, "Timestamp"=w609, "StudyName"=w607) -> (w608:T5)
                              n70 = Select(t=Hand."Left" ("Enum"), s=w612, f=Hand."Right" ("Enum")) -> (s? t:f=w614:T1)
                              "AssessmentMode" <- w611
                              "SubjectNr" <- w610
                              "DateTime" <- w609
                            }
                            frame #1 {
                              # "Set only after\nother vars\nwritten"
                              n71 = Send Notification "NotifyLog"(notification=w622, notifier=w621, error in (no error)=w619) -> (error out=w618:errorcluster)  [unwired: 1 out]
                              "SelectedHand" <- w620
                            }
                          }
                          n72 = TCP Write(connection ID=w596, data in="X", error in (no error)=w598, 9:-1 ("timeout ms (25000)")) -> (error out=w599:errorcluster)  [unwired: 2 out]
                        }
                        frame Error {
                        }
                      }
                    }
                    frame "Command" {
                      n73 = Unflatten From String(type=T17 {"EmergencyStop"=FALSE, "Start"=FALSE, "Restart"=FALSE, "FrontendStarted"=FALSE, "Close"=FALSE}, binary string=w634, data includes array or string size? (T)=FALSE, error in (no error)=w633) -> (value=w635:T17, error out=w632:errorcluster)  [unwired: 1 in, 1 out]
                      n74 = Unbundle By Name(w635) -> ("FrontendStarted"=w629:bool, "Start"=w628:bool, "EmergencyStop"=w627:bool, "Restart"=w626:bool, "Close"=w631:bool)
                      n75 = case shown="No Error" w632 {
                        selector: w632 -> [w643 w665]
                        tunnel: [w644 FALSE ("Close")] -> w630
                        tunnel: w631 -> [w645 _]
                        tunnel: w629 -> [w649 _]
                        tunnel: w628 -> [w648 _]
                        tunnel: w627 -> [w647 _]
                        tunnel: w626 -> [w646 _]
                        tunnel: w625 -> [w640 _]
                        tunnel: [w638 w665] -> w624
                        frame No Error {
                          # "Send\nReply"
                          n76 = flat-sequence {
                            tunnel: w649 -> [w652]
                            tunnel: w648 -> [w657]
                            tunnel: w647 -> [w651]
                            tunnel: w646 -> [w654]
                            tunnel: [w656] -> w644
                            tunnel: w645 -> [w656]
                            tunnel: [w655] -> w639
                            tunnel: w643 -> [w655]
                            frame #0 {
                              # "Only send reply for restart and stop\nonce tdms is closed\n(and state machine fully reset for restart)"
                              n77 = flat-sequence {
                                tunnel: w651 -> [w658]
                                tunnel: [w658] -> w650
                                frame #0 {
                                "StopSignal" <- w658
                                }
                              }
                              n78 = flat-sequence {
                                tunnel: w654 -> [w661]
                                tunnel: [w661] -> w653
                                frame #0 {
                                "RestartSignal" <- w661
                                }
                              }
                              n79 = case shown="True" w650 {
                                frame False {
                                }
                                frame True {
                                n80 = while {
                                stop <- w659 continue-if-true
                                n81 = local read "LogFileOpen"() -> (w659:bool)
                                n82 = Wait (ms)(milliseconds to wait=u32 30) -> ()  [unwired: 1 out]
                                }
                                }
                              }
                              n83 = case shown="True" w653 {
                                frame False {
                                }
                                frame True {
                                n84 = while {
                                stop <- w662 continue-if-true
                                n85 = local read "RestartSignal"() -> (w662:bool)
                                n86 = Wait (ms)(milliseconds to wait=u32 30) -> ()  [unwired: 1 out]
                                }
                                }
                              }
                              "FrontendStartedSignal" <- w652
                              "StartSignal" <- w657
                            }
                          }
                          n87 = TCP Write(connection ID=w640, data in="X", error in (no error)=w639, 9:-1 ("timeout ms (25000)")) -> (error out=w638:errorcluster)  [unwired: 2 out]
                        }
                        frame Error {
                        }
                      }
                    }
                    frame "Skip" {
                      # "Send\nReply"
                      n88 = flat-sequence {
                        tunnel: [w673] -> w668
                        tunnel: w667 -> [w673]
                        frame #0 {
                          "SkipSignal" <- TRUE ("SkipSignal")
                        }
                      }
                      n89 = TCP Write(connection ID=w666, data in="X", error in (no error)=w668, 9:-1 ("timeout ms (25000)")) -> (error out=w669:errorcluster)  [unwired: 2 out]
                    }
                    frame "BackendInfoReq" {
                      # "Send\nReply"
                      n90 = local read "Largest USB Partition Path"() -> (w676:path)
                      n91 = Path To String(path=w676) -> (string=w675:string)
                      n92 = Bundle By Name(cluster=T18 {"ProtocolVersion"=2, "DataPath"=""} ("Cluster"), "ProtocolVersion"=u16 2, "DataPath"=w675) -> (w678:T18)
                      n93 = Flatten To String(anything=w678, error in (no error)=w686) -> (data string=w680:string, error out=w685:errorcluster)  [unwired: 2 in, 1 out]
                      n94 = Concatenate Strings("Y" ("string"), w680) -> (w681:string)
                      n95 = TCP Write(connection ID=w684, data in=w681, error in (no error)=w685, 9:-1 ("timeout ms (25000)")) -> (connection ID out=w683:refnum<k5>, error out=w688:errorcluster)  [unwired: 1 out]
                    }
                  }
                  n96 = call <vilib>:"Clear Errors.vi"("error in (no error)"=w524, "specific error code to clear (0: all)"=56) -> ("error out"=w525:errorcluster)  [unwired: 4 in, 1 out]
                  n97 = flat-sequence "Stop Signal" {
                    tunnel: [w555] -> w530
                    tunnel: w525 -> [w555]
                    tunnel: w534 -> [w558]
                    tunnel: [w559] -> w533
                    frame #0 {
                      # "Reset connection\non error"
                      n98 = local read "StopRequested"() -> (w560:bool)
                      n99 = case shown="No Error" w555 {
                        tunnel: [FALSE TRUE] -> w556
                        frame No Error {
                        }
                        frame Error {
                        }
                      }
                      n100 = Or(x=w556, y=w558) -> (x .or. y?=w557:bool)
                      n101 = Or(x=w557, y=w560) -> (x .or. y?=w559:bool)
                    }
                  }
                  n102 = case shown="True" w533 {
                    tunnel: w522 -> [_ w554]
                    tunnel: w530 -> [w551 w553]
                    tunnel: [w551 w552] -> w526
                    frame False {
                    }
                    frame True {
                      n103 = TCP Close Connection "TCP Close"(connection ID=w554, error in (no error)=w553) -> (error out=w552:errorcluster)  [unwired: 1 in, 1 out]
                    }
                  }
                  "Error which lead\nto TCP close" <- w526
                }
              }
              frame Error {
                # "Probably timed out,\nbecause nobody connected\n-> try again in next iteration"
              }
            }
            n104 = flat-sequence "Stop Signal" {
              tunnel: [w508] -> w499
              tunnel: w500 -> [w506]
              frame #0 {
                n105 = local read "StopRequested"() -> (w508:bool)
                n106 = local write "Connected"(FALSE) -> ()
                n107 = local write "Remote IP"(u32 0 ("Remote IP")) -> ()
                "TCP Error" <- w506
              }
            }
          }
          n108 = node-c288() -> ()  [unwired: 1 in, 1 out]
        }
      }
      n109 = timed-loop {
        timing: w278 -> [_]
        timing-out: [_] -> w277
        tunnel: w276 -> [w704]
        tunnel: [w703] -> w264
        stop <- w701 stop-if-true
        # "UDP Socket"
        # "UDP Sending Loop"
        n110 = node-c288() -> ()  [unwired: 1 in, 1 out]
        n111 = call "UdpDataGlobal.vi"("Action"=UdpGlobalActions."Read") -> ("UDP Robot State"=w697:T41)  [unwired: 26 in]
        n112 = local read "Remote IP"() -> (w700:u32)
        n113 = Flatten To String(anything=w697, prepend array or string size? (T)=FALSE) -> (data string=w707:string, error out=w706:errorcluster)  [unwired: 2 in, 1 out]
        n114 = UDP Write(address=w700, port or service name="UDP Destination Port", connection ID=w704, data in=w707, 8:w706, 9:5 ("specific error code to clear (0: all)")) -> (error out=w705:errorcluster, 3:w703:refnum<k16>)
        n115 = flat-sequence "Stop Signal" {
          tunnel: w705 -> [w709]
          tunnel: [w710] -> w701
          tunnel: [w709] -> w699
          frame #0 {
            n116 = local read "StopRequested"() -> (w710:bool)
          }
        }
        n117 = node-c288() -> ()  [unwired: 1 in, 1 out]
        "UDP Error" <- w699
      }
      n118 = node-c288(w277) -> ()  [unwired: 1 out]
      n119 = node-c288(w271) -> ()  [unwired: 1 out]
      n120 = node-c288(60 ("Priority"), 1 ("Processor")) -> (w260:T11)  [unwired: 2 in]
      n121 = timed-sequence {
        timing: w260 -> [_]
        timing-out: [_] -> w259
        tunnel: w261 -> [w289]
        tunnel: w256 -> [w288]
        n122 = timed-flat-sequence {
          tunnel: w289 -> [w296]
          tunnel: w288 -> [w291]
          # "NewPatient Event Notifier"
          # "Buffer"
          # "Index"
          # "TDMS File"
          # "PatientData"
          # "GroupName"
          # "TDMS Logging"
          n123 = node-c288() -> ()  [unwired: 1 in, 1 out]
          n124 = local read "Largest USB Partition Path"() -> (w290:path)
          n125 = Initialize Array(0.0 ("element"), 50 ("dimension size"), 14 ("dimension size")) -> (w295:dbl[][])
          n126 = while {
            shift-right: [w318] -> _
            shift-left: TypeDef_TDMS_States."WaitingForCreate" ("TDMS States") -> [w317]
            shift-right: [w316] -> _
            shift-left: _ -> [w315]
            shift-right: [w314] -> _
            shift-left: _ -> [w313]
            shift-right: [w310] -> _
            shift-left: _ -> [w312]
            tunnel: w290 -> [w311]
            shift-right: [w307] -> _
            shift-left: string[] ["Time [s]", "Position [deg]", "Target Position [deg]", "Target state?", "Frontend Started", "Trial Nr", "Velocity [deg/s]", "Current [A]", "Starting position [deg]", "Voltage force [V]", "Force [N]", "Force filtered [N] ", "Velocity unfiltered", "ROM State 0-Active 1-Passive 2-Automatic"] -> [w309]
            tunnel: w296 -> [w306]
            shift-right: [w305] -> _
            shift-left: _ -> [w304]
            shift-right: [w302] -> _
            shift-left: w295 -> [w303]
            shift-right: [w301] -> _
            shift-left: _ -> [w300]
            tunnel: w291 -> [w299]
            stop <- w308 stop-if-true
            # "Stop when stop\nsignal is on\nand we are \nin a safe state"
            # "Logging"
            n127 = case shown="\"Create\"" w317 {
              selector: w317 -> [w324 _ w407 _ _ _]
              tunnel: [w322 w351 w422 TypeDef_TDMS_States."Close" ("TDMS States") w454 TypeDef_TDMS_States."WaitingForCreate" ("TDMS States")] -> w318
              tunnel: [w327 FALSE ("Button :: Stop") FALSE ("StopRequested") FALSE ("StopRequested") FALSE ("Button :: Stop") w475] -> w308
              tunnel: [w319 w339 w427 w439 w445 w473] -> w316
              tunnel: w315 -> [_ w343 w428 w440 w459 _]
              tunnel: [w328 w355 w429 w441 w458 _] -> w314
              tunnel: w313 -> [w328 _ w429 w441 w460 w478]
              tunnel: w312 -> [w330 _ w431 w442 w452 w476]
              tunnel: w311 -> [_ w338 _ _ _ _]
              tunnel: [w330 w354 w431 w442 w452 w476] -> w310
              tunnel: w309 -> [w329 w333 w430 w438 w449 w472]
              tunnel: [w329 w333 w430 w438 w449 w472] -> w307
              tunnel: w306 -> [_ w344 w426 _ _ _]
              tunnel: [w325 0 w414 0 0 0] -> w305
              tunnel: w304 -> [w325 _ w416 w434 _ _]
              tunnel: w303 -> [w331 w349 w421 w435 w450 w470]
              tunnel: [w331 w349 w419 w435 w450 w470] -> w302
              tunnel: [w332 w345 w404 w443 w447 w469] -> w301
              tunnel: w300 -> [_ w345 w404 w443 w447 w469]
              tunnel: w299 -> [w321 _ _ _ _ w468]
              frame "WaitingForCreate" {
                n128 = Wait on Notification "NewPatientSubmitted Event"(notifier=w321, timeout in ms (-1)=1000) -> (notification=w332:T5, timed out?=w320:bool, error out=w319:errorcluster)  [unwired: 2 in, 1 out]
                n129 = Select(t=w324, s=w320, f=TypeDef_TDMS_States."Create" ("TDMS States")) -> (s? t:f=w322:T9)
                n130 = local read "StopRequested"() -> (w327:bool)
              }
              frame "Create" {
                n131 = flat-sequence {
                  tunnel: w343 -> [w380]
                  tunnel: [w380] -> w342
                  frame #0 {
                    n132 = local write "LogFileOpen"(TRUE ("LogFileOpen")) -> ()
                  }
                }
                n133 = Unbundle By Name(w345) -> ("Timestamp"=w352:string, "Mode"=w353:T4, "StudyName"=w335:string, "Name"=w334:string, "Left"=w336:bool)
                n134 = Build Path(base path=w338, name or relative path=w335) -> (appended path=w337:path)
                n135 = case shown="\"PreciseReaching\"" w353 {
                  tunnel: ["Range Of Motion Task" ("name or relative path") "Force Task" ("name or relative path") "Precise Reaching Task" ("name or relative path") "Motor Task" ("name or relative path") "Sensorimotor Task" ("name or relative path") "Position Matching Task" ("name or relative path")] -> w369
                  frame "RangeOfMotion" {
                  }
                  frame "Force" {
                  }
                  frame "PreciseReaching" {
                  }
                  frame "Motor", Default {
                  }
                  frame "Sensorimotor" {
                  }
                  frame "PositionMatching" {
                  }
                }
                n136 = while {
                  shift-right: [w383] -> _
                  shift-left: w344 -> [w384]
                  shift-right: [w382] -> w341
                  shift-left: w342 -> [w382]
                  stop <- w385 stop-if-true
                  # "Clear Stale Data"
                  n137 = RT FIFO Read(0:w384) -> (8:w383:refnum<k33>, 10:w385:bool)  [unwired: 3 in, 3 out]
                }
                n138 = Build Path(base path=w337, name or relative path=w334) -> (appended path=w370:path)
                n139 = Select(t="Left Hand" ("name or relative path"), s=w336, f="Right Hand" ("name or relative path")) -> (s? t:f=w367:string)
                n140 = Build Path(base path=w370, name or relative path=w369) -> (appended path=w368:path)
                n141 = Build Path(base path=w368, name or relative path=w367) -> (appended path=w358:path)
                n142 = call <vilib>:"Check if File or Folder Exists.vi"("error in (no error)"=w341, "path"=w358) -> ("error out"=w361:errorcluster, "file or folder exists?"=w359:bool, "dup path"=w360:path)  [unwired: 7 in]
                n143 = case shown="False" w359 {
                  tunnel: w360 -> [w395 w396]
                  tunnel: [w394 w397] -> w364
                  tunnel: w361 -> [w393 w397]
                  tunnel: [w392 w396] -> w366
                  frame False {
                    n144 = Create Folder(path (use dialog)=w395, error in=w393) -> (created path=w392:path, error out=w394:errorcluster)  [unwired: 1 in, 1 out]
                  }
                  frame True {
                  }
                }
                n145 = flat-sequence {
                  tunnel: [w379] -> w348
                  tunnel: w340 -> [w374]
                  tunnel: [w374] -> w339
                  frame #0 {
                    n146 = local read "AssessmentFinished"() -> (w375:bool)
                    n147 = local read "StopRequested"() -> (w378:bool)
                    n148 = local read "RestartSignal"() -> (w377:bool)
                    n149 = Or(x=w377, y=w378) -> (x .or. y?=w376:bool)
                    n150 = Or(x=w376, y=w375) -> (x .or. y?=w379:bool)
                  }
                }
                n151 = Concatenate Strings(w352, ".tdms") -> (w357:string)
                n152 = Build Path(base path=w366, name or relative path=w357) -> (appended path=w362:path)
                n153 = TDMS Open(7:enum16{"1.0", "2.0"}."2.0" ("file format version (2.0)"), 8:w364, 10:T10."create" ("operation (0:open)"), 11:w362) -> (0:w340:errorcluster, 3:w355:refnum<k34>)  [unwired: 3 in]
                n154 = case shown="\"PreciseReaching\"" w353 {
                  tunnel: ["ROM Task" ("name or relative path") "Force Task" ("name or relative path") "Precise Reaching Task" ("name or relative path") "Motor Task" ("name or relative path") "Sensorimotor Task" ("name or relative path") "Position Matching" ("name or relative path")] -> w354
                  frame "RangeOfMotion" {
                  }
                  frame "Force" {
                  }
                  frame "PreciseReaching" {
                  }
                  frame "Motor", Default {
                  }
                  frame "Sensorimotor" {
                  }
                  frame "PositionMatching" {
                  }
                }
                n155 = Select(t=TypeDef_TDMS_States."Close" ("TDMS States"), s=w348, f=TypeDef_TDMS_States."Buffering" ("TDMS States")) -> (s? t:f=w351:T9)
              }
              frame "Buffering" {
                n156 = RT FIFO Read(0:w426, 2:10 ("timeout in ms (0)"), 3:w428) -> (9:w420:dbl[], 10:w417:bool, 11:w427:errorcluster)  [unwired: 1 in, 2 out]
                n157 = local read "AssessmentFinished"() -> (w412:bool)
                n158 = local read "StopRequested"() -> (w409:bool)
                n159 = local read "RestartSignal"() -> (w410:bool)
                n160 = Replace Array Subset(array=w421, new element=w420, index (row)=w416) -> (w419:dbl[][])  [unwired: 1 in]
                n161 = Or(x=w410, y=w409) -> (x .or. y?=w411:bool)
                n162 = Or(x=w411, y=w412) -> (x .or. y?=w408:bool)
                n163 = Select(t=TypeDef_TDMS_States."Flushing" ("TDMS States"), s=w408, f=w407) -> (s? t:f=w406:T9)
                n164 = Increment(x=w416) -> (x+1=w415:i32)
                n165 = Select(t=w416, s=w417, f=w415) -> (s? t:f=w414:i32)
                n166 = Equal?(x=50, y=w414) -> (x = y?=w424:bool)
                n167 = Select(t=TypeDef_TDMS_States."Write" ("TDMS States"), s=w424, f=w406) -> (s? t:f=w422:T9)
              }
              frame "Flushing" {
                n168 = Array Subset(array=w435, length (row)=w434) -> (w433:dbl[][])  [unwired: 3 in]
                n169 = TDMS Write(0:w441, 1:enum16{"decimated", "interleaved"}."interleaved" ("data layout (0:decimated)"), 5:w442, 7:w438, 9:w433, 11:w440) -> (15:w439:errorcluster)  [unwired: 3 out]
              }
              frame "Write" {
                n170 = TDMS Write(0:w460, 1:enum16{"decimated", "interleaved"}."interleaved" ("data layout (0:decimated)"), 5:w452, 7:w449, 9:w450, 11:w459) -> (4:w458:refnum<k34>, 15:w446:errorcluster)  [unwired: 2 out]
                n171 = flat-sequence {
                  tunnel: [w462] -> w451
                  tunnel: w446 -> [w461]
                  tunnel: [w461] -> w445
                  frame #0 {
                    n172 = local read "AssessmentFinished"() -> (w466:bool)
                    n173 = local read "StopRequested"() -> (w463:bool)
                    n174 = local read "RestartSignal"() -> (w464:bool)
                    n175 = Or(x=w464, y=w463) -> (x .or. y?=w465:bool)
                    n176 = Or(x=w465, y=w466) -> (x .or. y?=w462:bool)
                  }
                }
                n177 = Select(t=TypeDef_TDMS_States."Close" ("TDMS States"), s=w451, f=TypeDef_TDMS_States."Buffering" ("TDMS States")) -> (s? t:f=w454:T9)
              }
              frame "Close" {
                # "Ensure notifier buffer is empty before going back to WaitingForCreate"
                n178 = Cancel Notification(0:w468) -> (11:w467:errorcluster)  [unwired: 1 in, 2 out]
                n179 = TDMS Close(8:w467, 11:w478) -> (0:w474:errorcluster)  [unwired: 1 out]
                n180 = flat-sequence {
                  tunnel: w474 -> [w480]
                  tunnel: [w480] -> w473
                  frame #0 {
                    # "Unset after file was closed"
                    n181 = local write "LogFileOpen"(FALSE ("LogFileOpen")) -> ()
                  }
                }
                n182 = local read "StopRequested"() -> (w475:bool)
              }
            }
          }
          n183 = node-c288() -> ()  [unwired: 1 in, 1 out]
        }
      }
      n184 = call "safety_range.vi"() -> ("Safety Range"=w250:dbl)  [unwired: 2 in]
      n185 = timed-loop "Main Control Loop" {
        timing: w287 -> [_]
        timing-out: [_] -> w286
        tunnel: w285 -> [w767]
        tunnel: [w766] -> w249
        shift-right: [w740] -> _
        shift-left: w280 -> [w725]
        tunnel: w282 -> [w760]
        shift-right: [w727] -> _
        shift-left: w262 -> [w728]
        shift-right: [w757] -> _
        shift-left: w279 -> [w743]
        shift-right: [w736] -> _
        shift-left: w266 -> [w739]
        shift-right: [w733] -> _
        shift-left: w265 -> [w734]
        tunnel: w261 -> [w726]
        tunnel: w254 -> [w724]
        tunnel: w252 -> [w723]
        tunnel: w253 -> [w722]
        tunnel: w251 -> [w721]
        tunnel: w250 -> [w720]
        tunnel: w245 -> [w719]
        stop <- w762 stop-if-true
        # "Assessment Mode"
        # "Phase Trial Count"
        # "Task State"
        # "Trial Nr"
        # "Loop Count"
        n186 = node-c288() -> (w761:bool, w768:i64)  [unwired: 1 in, 14 out]
        n187 = flat-sequence {
          tunnel: w768 -> [w802]
          tunnel: [w798] -> w756
          tunnel: w725 -> [w798]
          tunnel: [w782] -> w754
          tunnel: [w814] -> w752
          tunnel: [w822] -> w750
          tunnel: w761 -> [w829]
          tunnel: w760 -> [w827]
          tunnel: [w823] -> w748
          tunnel: w728 -> [w823]
          tunnel: [w771] -> w744
          tunnel: w743 -> [w771]
          tunnel: w739 -> [w821]
          tunnel: [w821] -> w738
          tunnel: [w809] -> w735
          tunnel: w734 -> [w809]
          tunnel: [w782] -> w730
          tunnel: w726 -> [w808]
          tunnel: w724 -> [w787]
          tunnel: w723 -> [w786]
          tunnel: w722 -> [w785]
          tunnel: w721 -> [w784]
          tunnel: w719 -> [w783]
          tunnel: w756 -> [w845]
          tunnel: [w845] -> w755
          tunnel: w754 -> [w849]
          tunnel: [w849] -> w753
          tunnel: w752 -> [w846]
          tunnel: [w846] -> w751
          tunnel: w750 -> [w848]
          tunnel: [w848] -> w749
          tunnel: w748 -> [w847]
          tunnel: [w847] -> w747
          tunnel: [w840] -> w746
          tunnel: [w839] -> w745
          tunnel: w744 -> [w837]
          tunnel: [w837] -> w742
          tunnel: [w842] -> w741
          tunnel: w738 -> [w844]
          tunnel: [w843] -> w737
          tunnel: w735 -> [w841]
          tunnel: [w838] -> w731
          tunnel: w730 -> [w838]
          tunnel: [w892] -> w765
          tunnel: w755 -> [w888]
          tunnel: [w882] -> w764
          tunnel: [w881] -> w763
          tunnel: w753 -> [w881]
          tunnel: w751 -> [w890]
          tunnel: w749 -> [w891]
          tunnel: w747 -> [w884]
          tunnel: [w876] -> w759
          tunnel: [w889] -> w758
          tunnel: w746 -> [w886]
          tunnel: w745 -> [w887]
          tunnel: w742 -> [w885]
          tunnel: w741 -> [w883]
          tunnel: w737 -> [w878]
          tunnel: [w879] -> w732
          tunnel: w731 -> [w880]
          tunnel: [w877] -> w729
          tunnel: w767 -> [w1491]
          tunnel: w765 -> [w1478]
          tunnel: w764 -> [w1487]
          tunnel: w763 -> [w1489]
          tunnel: w759 -> [w1488]
          tunnel: w758 -> [w1482]
          tunnel: [w1490] -> w766
          tunnel: [w1474] -> w740
          tunnel: [w1485] -> w762
          tunnel: [w1488] -> w727
          tunnel: [w1482] -> w757
          tunnel: [w1481] -> w736
          tunnel: [w1480] -> w733
          tunnel: w732 -> [w1480]
          tunnel: w729 -> [w1481]
          tunnel: w720 -> [w1467]
          frame #0 {
            # "pos   | v|c| vf |f|ff| vuf"
            # "Writing Data to Log Queue (rt fifo)"
            # "Position"
            # "Assessment Mode"
            # "Phase Trial Count"
            # "Force Sensor"
            # "Motor Current Monitor"
            # "Tachometer"
            # "Trial Nr"
            # "Task State"
            # "Loop Count"
            # "Position"
            # "Velocity"
            # "Period"
            # "Encoder"
            # "Period (s)"
            # "Calculate position/velocity etc"
            n188 = local read "AssessmentFinished"() -> (w774:bool)
            n189 = call "Tick Count"() -> ("Tick Count(mSec)"=w828:u32)
            n190 = To Double Precision Float(number=w802) -> (double precision float=w803:dbl)
            n191 = To Double Precision Float(number=1000000) -> (double precision float=w801:dbl)
            n192 = local read "LogFileOpen"() -> (w772:bool)
            n193 = Divide(x=w803, y=w801) -> (x/y=w822:dbl)
            n194 = Subtract(x=w828, y=w827) -> (x-y=w805:u32)
            n195 = call <vilib>:"Read.vi"("Encoder Ref In"=w787) -> ("Counter Value"=w836:i32)  [unwired: 6 in, 4 out]
            n196 = call <vilib>:"Read.vi"("AI Ref In"=w784) -> ("Values"=w834:dbl[])  [unwired: 8 in, 2 out]
            n197 = call <vilib>:"Read.vi"("AI Ref In"=w786) -> ("Values"=w832:dbl[])  [unwired: 8 in, 2 out]
            n198 = call <vilib>:"Read.vi"("AI Ref In"=w785) -> ("Values"=w825:dbl[])  [unwired: 8 in, 2 out]
            n199 = Not(x=w772) -> (.not. x?=w773:bool)
            n200 = To Double Precision Float(number=w805) -> (double precision float=w807:dbl)
            n201 = To Double Precision Float(number=u32 1000 ("y")) -> (double precision float=w806:dbl)
            n202 = And(x=w774, y=w773) -> (x .and. y?=w770:bool)
            n203 = Index Array(array=w834, index=0) -> (element=w833:dbl)
            n204 = Index Array(array=w832, index=0) -> (element=w830:dbl)
            n205 = Index Array(array=w825, index=0) -> (element=w812:dbl)
            "Voltage force" <- w812
            n206 = Divide(x=w807, y=w806) -> (x/y=w775:dbl)
            "Time (s)" <- w775
            n207 = call "TF_Encoder2Position.vi"("Counter Value"=w836) -> ("Position [deg]"=w782:dbl)  [unwired: 4 in]
            "Position [deg]" <- w782
            n208 = call "TF_Tacho2VelocityV2.vi"("Motor Velocity Tacho Value [V]"=w833) -> ("Motor Velocity Tacho [deg/s]"=w811:dbl)  [unwired: 4 in]
            "Velocity unfiltered [deg/s]" <- w811
            n209 = call "TF_MotorCurrentInput.vi"("Motor Current Monitor Value [V]"=w830) -> ("Current [A]"=w813:dbl)
            "Current [A]" <- w813
            n210 = call "TF_StrainGauge2ForceV2.vi"("Strain Gauge Value [V]"=w812) -> ("Force [N]"=w789:dbl)  [unwired: 4 in]
            n211 = local read "FrontendStartedSignal"() -> (w817:bool)
            n212 = Subtract(x=w789, y=w783) -> (x-y=w788:dbl)
            "Force" <- w788
            n213 = local read "Target Position [deg]"() -> (w780:dbl)
            n214 = local read "Starting position"() -> (w781:dbl)
            n215 = local read "Target state?"() -> (w777:bool)
            n216 = local read "ROM State"() -> (w776:T2)
            n217 = Reciprocal(x=w822) -> (1/x=w797:dbl)
            n218 = Reciprocal(x=w822) -> (1/x=w793:dbl)
            n219 = Boolean To (0,1)(Boolean=w777) -> (0, 1=w819:i16)
            n220 = Boolean To (0,1)(Boolean=w817) -> (0, 1=w799:i16)
            n221 = call <vilib>:"Butterworth Filter PtByPt.vi"("order"=1, "filter type"=Filter_Passband_Type."Lowpass", "low cutoff freq: fl"=20.0, "sampling freq: fs"=w797, "x"=w811) -> ("Filtered x"=w814:dbl)  [unwired: 4 in, 1 out]
            "Velocity [deg/s]" <- w814
            n222 = To Double Precision Float(number=w819) -> (double precision float=w818:dbl)
            n223 = To Double Precision Float(number=w799) -> (double precision float=w816:dbl)
            n224 = First Call?() -> (First Call?: T/F=w824:bool)
            n225 = call <vilib>:"Butterworth Filter PtByPt.vi"("initialize"=w824, "order"=1, "filter type"=Filter_Passband_Type."Lowpass", "low cutoff freq: fl"=20.0, "sampling freq: fs"=w793, "x"=w788) -> ("Filtered x"=w779:dbl)  [unwired: 3 in, 1 out]
            "Force filtered" <- w779
            n226 = To Double Precision Float(number=w771) -> (double precision float=w815:dbl)
            n227 = To Double Precision Float(number=w776) -> (double precision float=w810:dbl)
            n228 = local read "Flexion"() -> (w778:bool)
            n229 = Build Array(w775, w782, w780, w818, w816, w815, w814, w813, w781, w812, w788, w779, w811, w810) -> (w820:dbl[])
            n230 = RT FIFO Write(0:w808, 1:w820) -> ()  [unwired: 3 in, 4 out]
            n231 = call "UdpDataGlobal.vi"("Position"=w782, "Starting Position"=w781, "Target Position"=w780, "Force"=w779, "TargetState"=w777, "RomState"=w776, "Time"=w775, "Finished"=w770, "Flexion"=w778, "Trial Nr"=w771, "Action"=UdpGlobalActions."Write") -> ()  [unwired: 16 in, 1 out]
            "Finished late?" <- w829
          }
          frame #1 {
            # "Reading Selection and Reset"
            n232 = case "Hand And Mode Selection" shown="\"Hand choice\"" w845 {
              tunnel: [TRUE w854] -> w839
              tunnel: [w853 w860] -> w842
              tunnel: w844 -> [w852 w858]
              tunnel: [w852 w857] -> w843
              tunnel: [w851 w856] -> w840
              tunnel: w841 -> [w851 w855]
              frame Default {
                n233 = local read "LeftHand"() -> (w853:bool)
              }
              frame "Hand choice" {
                n234 = local read "SelectedHand"() -> (w859:T1)
                n235 = case shown="Default" w859 {
                  selector: w859 -> [_ w872]
                  tunnel: [FALSE TRUE] -> w854
                  tunnel: [_ w865] -> w860
                  tunnel: w858 -> [w862 _]
                  tunnel: [w862 w869] -> w857
                  tunnel: [w861 w868] -> w856
                  tunnel: w855 -> [w861 _]
                  frame "None" {
                  }
                  frame Default {
                    n236 = local read "AssessmentMode"() -> (w868:T4)
                    n237 = local read "Phase Trial Count"() -> (w866:i16)
                    n238 = call "IsFirstIteration.vi"("Trial Nr"=i16 -1) -> ()  [unwired: 2 in, 1 out]
                    n239 = local write "ROM State"(ROM_States."Active" ("Enum")) -> ()
                    n240 = Equal?(x=w872, y=Hand."Left" ("Enum")) -> (x = y?=w865:bool)
                    "LeftHand" <- w865
                    n241 = case shown="\"PositionMatching\"" w868 {
                      tunnel: [i16 1 i16 2] -> w867
                      frame Default {
                      }
                      frame "PositionMatching" {
                      }
                    }
                    n242 = Max & Min(x=w867, y=w866) -> (max(x,y)=w869:i16)  [unwired: 1 out]
                  }
                }
              }
            }
          }
          frame #2 {
            # "Task State"
            # "Position [deg]"
            # "Phase Trial Count"
            # "StartAssessment"
            # "Velocity"
            # "Assessment Mode"
            # "Loop Count"
            # "Period"
            # "Position [deg]"
            # "Left Hand?"
            # "Trial Nr"
            # "State Machine"
            n243 = case shown="\"Resetting\"" w888 {
              selector: w888 -> [w901 w913 _ _ w1451]
              tunnel: [w900 w905 w1147 Main_States."WaitingForRestart" ("Task states") w1450] -> w892
              tunnel: [0.0 ("u") w917 w1162 0.0 ("u") 0.0 ("u")] -> w882
              tunnel: w880 -> [_ w915 w1154 _ _]
              tunnel: w891 -> [_ w921 w1163 _ _]
              tunnel: w890 -> [_ w920 w1158 _ _]
              tunnel: w884 -> [_ _ w1152 _ _]
              tunnel: [0 0 w1150 0 0] -> w876
              tunnel: [w897 w902 w1165 w1443 w1456] -> w889
              tunnel: w885 -> [_ w911 w1166 w1443 w1456]
              tunnel: w887 -> [w893 _ _ _ _]
              tunnel: w883 -> [_ w912 w1151 _ _]
              tunnel: w886 -> [w894 w907 w1155 w1446 w1457]
              tunnel: w878 -> [w895 w908 w1157 w1447 w1458]
              tunnel: [w895 w904 w1156 w1447 w1458] -> w877
              tunnel: [w894 w906 w1155 w1446 w1457] -> w879
              tunnel: w881 -> [_ _ w1153 _ _]
              frame "Hand choice", Default {
                w897 = i16 1  # Trial Nr
                # "Current Task State"
                n244 = Select(t=Main_States."Start" ("Task states"), s=w893, f=w901) -> (s? t:f=w900:T3)
              }
              frame "Start" {
                # "Trial Nr [OUT]"
                # "Phase Trial Count"
                # "Assessment Mode"
                # "Trial Nr [IN]"
                # "Starting Position"
                # "Position"
                n245 = case "Calculating starting Position and Target Arrays" shown="\"PreciseReaching\"" w907 {
                  selector: w907 -> [_ _ w1096 w1116 _ w1136]
                  tunnel: [w1048 0.0 ("f") w1082 w1108 w1129 w1137] -> w914
                  tunnel: w911 -> [w1045 w1071 w1086 w1112 w1127 w1133]
                  tunnel: w912 -> [w1047 _ w1083 w1109 w1130 w1135]
                  tunnel: w908 -> [w1046 w1073 w1081 w1107 w1128 w1132]
                  tunnel: [w1046 w1073 w1081 w1107 w1128 w1132] -> w904
                  tunnel: [w1045 w1071 w1086 w1112 w1127 w1133] -> w903
                  frame "RangeOfMotion" {
                    n246 = local read "ROM State"() -> (w1049:T2)
                    n247 = case shown="\"Active\", \"Passive\", Default" w1049 {
                      tunnel: [w1051 w1067] -> w1048
                      tunnel: w1047 -> [w1052 w1070]
                      frame "AutomaticPassive" {
                        # "Determine middle between max and\nmin range to start sinewave from"
                        # "If limit is above 82 the arm can crash\ninto the end of the guidance if the \npatient has a big range of motion"
                        n248 = local read "ROM max"() -> (w1054:dbl)
                        n249 = call "angle_limit.vi"() -> ("LimitAngle"=w1050:dbl)  [unwired: 2 in]
                        n250 = case "Limit max Angle" shown="False" w1052 {
                          tunnel: w1054 -> [w1058 w1065]
                          tunnel: [w1061 w1064] -> w1053
                          tunnel: w1050 -> [w1060 w1063]
                          frame False {
                            n251 = Negate(x=w1060) -> (-x=w1059:dbl)
                            n252 = Greater?(x=w1058, y=w1059) -> (0:w1062:bool)
                            n253 = Select(t=w1058, s=w1062, f=w1059) -> (s? t:f=w1061:dbl)
                          }
                          frame True {
                            n254 = Less?(x=w1065, y=w1063) -> (x < y?=w1066:bool)
                            n255 = Select(t=w1065, s=w1066, f=w1063) -> (s? t:f=w1064:dbl)
                          }
                        }
                        n256 = local write "ROM max"(w1053) -> ()
                        n257 = local read "ROM min"() -> (w1055:dbl)
                        n258 = Add(x=w1053, y=w1055) -> (x+y=w1056:dbl)
                        n259 = Divide(x=w1056, y=2.0) -> (x/y=w1051:dbl)
                        "Zero Position" <- w1051
                        n260 = local write "Starting position"(w1051) -> ()
                      }
                      frame "Active", "Passive", Default {
                        w1069 = 30.0
                        n261 = Negate(x=w1069) -> (-x=w1068:dbl)
                        n262 = Select(t=w1069, s=w1070, f=w1068) -> (s? t:f=w1067:dbl)
                      }
                    }
                  }
                  frame "Force" {
                    # "Only write if the trial nr\nhas changed and at the \nfirst iteration\n(due to performace reasons)"
                    n263 = feedback-in #1(w1071) -> ()
                    n264 = feedback #1(i16 -1 ("Trial Nr")) -> (w1072:i16)
                    n265 = Not Equal?(x=w1072, y=w1071) -> (x != y?=w1075:bool)
                    n266 = case "Set Flexion Flag" shown="True" w1075 {
                      tunnel: w1071 -> [_ w1078]
                      tunnel: w1073 -> [_ w1077]
                      frame False {
                      }
                      frame True {
                        n267 = Less Or Equal?(x=w1078, y=w1077) -> (x <= y?=→"Flexion":bool)
                      }
                    }
                  }
                  frame "Motor" {
                    # "Generate random target array"
                    # "Left Hand?"
                    # "Flexion?"
                    # "Choose the starting position based on the target position"
                    # "Generate Target Array on first call"
                    n268 = call "IsFirstIteration.vi"("Left Hand"=w1083, "AssessmentMode"=w1096, "Trial Nr"=w1086) -> ("Is First Iteration"=w1095:bool)
                    n269 = To Long Integer(number=w1081) -> (32bit integer=w1080:i32)
                    n270 = case shown="True" w1095 {
                      tunnel: [w1098 w1101] -> w1097
                      tunnel: w1083 -> [_ w1102]
                      tunnel: w1080 -> [_ w1099]
                      frame False {
                        n271 = local read "Target Array"() -> (w1098:dbl[])
                      }
                      frame True {
                        w1104 = dbl[] [30.0, 70.0]
                        n272 = Negate(x=w1104) -> (-x=w1103:dbl[])
                        n273 = Select(t=w1104, s=w1102, f=w1103) -> (s? t:f=w1100:dbl[])
                        n274 = call "create_target_abs_v2.vi"("NumRepetitions"=w1099, "Inputs"=w1100) -> ("Target Array"=w1101:dbl[])  [unwired: 9 in]
                        "Target Array" <- w1101
                      }
                    }
                    n275 = Decrement(x=w1086) -> (x-1=w1085:i16)
                    n276 = To Long Integer(number=w1085) -> (32bit integer=w1084:i32)
                    n277 = Index Array(array=w1097, index=w1084) -> (element=w1087:dbl)
                    n278 = local write "Target Position [deg]"(w1087) -> ()
                    n279 = Absolute Value(x=w1087) -> (abs(x)=w1093:dbl)
                    n280 = Less?(x=w1093, y=45.0) -> (x < y?=w1092:bool)
                    n281 = Select(t=70.0 ("y"), s=w1092, f=30.0 ("y")) -> (s? t:f=w1088:dbl)
                    n282 = Negate(x=w1088) -> (-x=w1089:dbl)
                    n283 = Select(t=w1088, s=w1083, f=w1089) -> (s? t:f=w1082:dbl)
                    n284 = local write "Starting position"(w1082) -> ()
                  }
                  frame "PreciseReaching" {
                    w1105 = 30.0
                    # "Generate random target array"
                    # "Generate Target Array on first call"
                    n285 = call "IsFirstIteration.vi"("Left Hand"=w1109, "AssessmentMode"=w1116, "Trial Nr"=w1112) -> ("Is First Iteration"=w1115:bool)
                    n286 = Negate(x=w1105) -> (-x=w1114:dbl)
                    n287 = Select(t=w1105, s=w1109, f=w1114) -> (s? t:f=w1108:dbl)
                    n288 = To Long Integer(number=w1107) -> (32bit integer=w1106:i32)
                    n289 = case shown="True" w1115 {
                      tunnel: [w1118 w1119] -> w1117
                      tunnel: w1109 -> [_ w1122]
                      tunnel: w1106 -> [_ w1120]
                      frame False {
                        n290 = local read "Target Array"() -> (w1118:dbl[])
                      }
                      frame True {
                        w1124 = dbl[] [50.0, 70.0]
                        n291 = Negate(x=w1124) -> (-x=w1123:dbl[])
                        n292 = Select(t=w1124, s=w1122, f=w1123) -> (s? t:f=w1121:dbl[])
                        n293 = call "create_target_abs_v2.vi"("NumRepetitions"=w1120, "Inputs"=w1121) -> ("Target Array"=w1119:dbl[])  [unwired: 9 in]
                        n294 = local write "Target Array"(w1119) -> ()
                      }
                    }
                    n295 = local write "Starting position"(w1108) -> ()
                    n296 = Decrement(x=w1112) -> (x-1=w1111:i16)
                    n297 = To Long Integer(number=w1111) -> (32bit integer=w1110:i32)
                    n298 = Index Array(array=w1117, index=w1110) -> (element=w1113:dbl)
                    n299 = local write "Target Position [deg]"(w1113) -> ()
                  }
                  frame "Sensorimotor" {
                    w1126 = 45.0
                    n300 = Negate(x=w1126) -> (-x=w1125:dbl)
                    n301 = Select(t=w1126, s=w1130, f=w1125) -> (s? t:f=w1129:dbl)
                    n302 = local write "Starting position"(w1129) -> ()
                    n303 = local write "Target Position [deg]"(w1129) -> ()
                  }
                  frame "PositionMatching" {
                    n304 = call "IsFirstIteration.vi"("Left Hand"=w1135, "AssessmentMode"=w1136, "Trial Nr"=w1133) -> ("Is First Iteration"=w1134:bool)
                    n305 = To Long Integer(number=w1132) -> (32bit integer=w1131:i32)
                    n306 = case shown="True" w1134 {
                      tunnel: w1135 -> [_ w1141]
                      tunnel: [w1138 w1140] -> w1137
                      tunnel: w1131 -> [_ w1139]
                      frame False {
                        n307 = local read "Starting position"() -> (w1138:dbl)
                      }
                      frame True {
                        w1143 = 30.0  # Max Range
                        w1142 = 10.0  # Min Range
                        w1146 = 30.0 ("t")
                        n308 = Negate(x=w1146) -> (-x=w1145:dbl)
                        n309 = Select(t=w1146, s=w1141, f=w1145) -> (s? t:f=w1140:dbl)
                        n310 = call "GenerateTargetArrayForRange_v2.vi"("Max Range"=w1143, "Min Range"=w1142, "Left Hand"=w1141, "Num Steps (Inclusive)"=w1139, "Starting Position"=w1140) -> ("Target Array"=w1144:dbl[])
                        n311 = local write "Starting position"(w1140) -> ()
                        n312 = local write "Target Array"(w1144) -> ()
                      }
                    }
                  }
                }
                n313 = local read "StartSignal"() -> (w910:bool)
                n314 = Variant To Flattened String(Variant=w910) -> (data string=w919:string)  [unwired: 1 out]
                n315 = First Call?() -> (First Call?: T/F=w918:bool)
                n316 = call "Value Has Changed String PtByPt.vi"("input data point"=w919, "initialize"=w918) -> ("has changed"=w916:bool)  [unwired: 1 out]
                n317 = case shown="True" w910 {
                  tunnel: [w928 w961] -> w905
                  tunnel: w921 -> [_ w967]
                  tunnel: w920 -> [_ w966]
                  tunnel: [0.0 ("u") w965] -> w917
                  tunnel: w916 -> [_ w964]
                  tunnel: w915 -> [_ w959]
                  tunnel: w914 -> [_ w958]
                  tunnel: w913 -> [w929 _]
                  tunnel: w907 -> [w927 w957]
                  tunnel: [w926 w956] -> w906
                  tunnel: w903 -> [w924 w955]
                  tunnel: w904 -> [w923 _]
                  tunnel: [w922 w955] -> w902
                  frame False {
                    n318 = local read "SkipSignal"() -> (w925:bool)
                    n319 = case shown="True" w925 {
                      tunnel: w929 -> [w933 _]
                      tunnel: [w933 w940] -> w928
                      tunnel: w927 -> [w932 w939]
                      tunnel: [w932 w939] -> w926
                      tunnel: w924 -> [w931 w938]
                      tunnel: w923 -> [_ w937]
                      tunnel: [w931 w934] -> w922
                      frame False {
                      }
                      frame True {
                        n320 = case shown="\"Sensorimotor\"" w939 {
                          tunnel: w938 -> [w944 w950]
                          tunnel: w937 -> [_ w951]
                          tunnel: [FALSE w948] -> w936
                          tunnel: [w944 w953] -> w934
                          frame Default {
                          }
                          frame "Sensorimotor" {
                            n321 = Quotient & Remainder(x=w950, y=w951) -> (x-y*floor(x/y)=w952:i16)  [unwired: 1 out]
                            n322 = Increment(x=w951) -> (x+1=w946:i16)
                            n323 = Equal? "firstTrialOfPhase?"(x=i16 1, y=w952) -> (x = y?=w949:bool)
                            n324 = Greater? "afterFirstInLastPhase?"(x=w950, y=w946) -> (0:w948:bool)
                            n325 = Or(x=w949, y=w948) -> (x .or. y?=w947:bool)
                            n326 = Select(t=w950, s=w947, f=w946) -> (s? t:f=w953:i16)
                          }
                        }
                        n327 = case shown="True" w936 {
                          tunnel: [Main_States."Start" ("Task states") Main_States."Resetting" ("Task states")] -> w940
                          frame False {
                            # "Skip Phase"
                          }
                          frame True {
                            # "Skip to Finished"
                            n328 = local write "AssessmentFinished"(TRUE ("AssessmentFinished")) -> ()
                          }
                        }
                        n329 = local write "SkipSignal"(FALSE ("SkipSignal")) -> ()
                      }
                    }
                  }
                  frame True {
                    # "In Position Matching TargetState is set later"
                    n330 = case "Move to the Starting Position" shown="Default" w957 {
                      tunnel: w959 -> [_ w1021]
                      tunnel: w967 -> [_ w1018]
                      tunnel: w966 -> [_ w1019]
                      tunnel: w964 -> [w974 w1033]
                      tunnel: [0.0 w1022] -> w965
                      tunnel: w958 -> [_ w1034]
                      tunnel: [w975 w1032] -> w960
                      frame "Force" {
                        # "Nonblocking wait for realtime systems.\nLoop will keep running until the timer\nhas reached the set amount.\nThis wait is for the patient to prepare"
                        n331 = feedback #2(TRUE ("done")) -> (w973:bool)
                        n332 = Or(x=w974, y=w973) -> (x .or. y?=w972:bool)
                        n333 = xnode "Elapsed Timer"("reset"=w972) -> ("elapsed time (ms)"=w977:i32)  [unwired: 2 in, 1 out]
                        n334 = Greater Or Equal?(x=w977, y=3000 ("milliseconds to wait")) -> (x >= y?=w975:bool)
                        n335 = feedback-in #2(w975) -> ()
                      }
                      frame Default {
                        w1023 = T42 {"output high"=5.0, "output low"=-5.0}  # Output range
                        n336 = feedback #3(TRUE ("profile complete?")) -> (w1031:bool)
                        n337 = Or(x=w1033, y=w1031) -> (x .or. y?=w1037:bool)
                        n338 = feedback #4() -> (w1036:cluster{"time (s)":dbl, "setpoint":dbl}[])  [unwired: 1 in]
                        n339 = case shown="True" w1037 {
                          tunnel: [w1038 w1043] -> w1035
                          tunnel: w1021 -> [_ w1040]
                          tunnel: w1036 -> [w1038 _]
                          tunnel: w1034 -> [_ w1041]
                          frame False {
                          }
                          frame True {
                            n340 = call "motion_create_minimum_jerk.vi"("Initial Position"=w1040, "Final Position"=w1041, "Initial Time [s]"=0.0, "Final Time [s]"=3.0, "Delta Time [s]"=0.01) -> ("Profile"=w1043:cluster{"time (s)":dbl, "setpoint":dbl}[])  [unwired: 10 in]
                          }
                        }
                        n341 = feedback-in #4(w1035) -> ()
                        n342 = call <vilib>:"PID Setpoint Profile.vi"("reinitialize? (F)"=w1037, "setpoint profile"=w1035) -> ("profile complete?"=w1032:bool, "setpoint"=w1020:dbl)  [unwired: 4 in, 2 out]
                        n343 = feedback-in #3(w1032) -> ()
                        n344 = call "min_jerk_params.vi"() -> ("Gains"=w1024:T43, "Non-linear gain"=w1025:T44, "D-Part variable"=w1026:T46, "Velocity estimate dy/dt"=w1027:T47, "Anti reset windup"=w1028:bool, "I-Part error band"=w1029:dbl)  [unwired: 14 in]
                        n345 = call "ENPIDv2.vi"("Gains"=w1024, "Non-linear gain"=w1025, "D-Part variable"=w1026, "Velocity estimate dy/dt"=w1027, "Anti reset windup"=w1028, "I-Part error band"=w1029, "Output range"=w1023, "y"=w1021, "r"=w1020, "dy/dt"=w1019, "dt (s)"=w1018) -> ("u"=w1022:dbl)  [unwired: 7 in, 1 out]
                      }
                    }
                    n346 = case shown="Default" w957 {
                      selector: w957 -> [w969 w970]
                      tunnel: w960 -> [_ w971]
                      tunnel: [w969 w970] -> w956
                      frame "PositionMatching" {
                      }
                      frame Default {
                        n347 = local write "Target state?"(w971) -> ()
                      }
                    }
                    n348 = case shown="True" w960 {
                      frame False {
                      }
                      frame True {
                        w968 = FALSE
                        n349 = local write "StartSignal"(w968) -> ()
                        n350 = local write "SkipSignal"(w968) -> ()
                      }
                    }
                    n351 = Select(t=Main_States."Show target" ("Task states"), s=w960, f=Main_States."Start" ("Task states")) -> (s? t:f=w961:T3)
                  }
                }
              }
              frame "Show target" {
                # "Loop Count"
                # "Selects next state depending\non if a trial is finished and\nif the max amount of trials\nhas been reached"
                # "Trial Finished"
                # "Max Trial reached"
                # "Phase Trial Count"
                # "Current"
                # "Current Setpoint"
                # "PID Finished"
                # "Loop Count"
                # "Trial Nr"
                n352 = case shown="\"Motor\", Default" w1155 {
                  tunnel: w1152 -> [w1179 w1312 _ w1334 w1373 w1410]
                  tunnel: w1166 -> [w1184 w1301 w1317 w1331 w1347 w1418]
                  tunnel: [w1183 w1307 w1323 w1339 w1379 w1408] -> w1165
                  tunnel: [w1182 w1310 w1325 w1341 w1382 w1420] -> w1164
                  tunnel: [w1181 w1308 w1318 w1332 w1363 w1405] -> w1148
                  tunnel: w1154 -> [w1188 _ _ _ _ w1390]
                  tunnel: w1163 -> [w1187 _ _ _ _ w1397]
                  tunnel: w1158 -> [w1186 _ _ _ _ w1393]
                  tunnel: [w1176 TRUE ("profile complete?") TRUE ("profile complete?") TRUE ("profile complete?") TRUE ("profile complete?") w1391] -> w1161
                  tunnel: [w1180 0.0 ("u") 0.0 ("u") 0.0 ("u") 0.0 ("u") w1392] -> w1160
                  tunnel: w1157 -> [w1178 w1302 w1319 w1335 w1384 w1407]
                  tunnel: [w1177 w1302 w1319 w1335 w1384 w1407] -> w1156
                  tunnel: w1151 -> [w1175 _ _ _ w1348 _]
                  frame "RangeOfMotion" {
                    # "Left Hand?"
                    n353 = local read "ROM State"() -> (w1185:T2)
                    n354 = case shown="\"AutomaticPassive\"" w1185 {
                      selector: w1185 -> [w1198 _]
                      tunnel: w1188 -> [w1199 w1250]
                      tunnel: w1187 -> [_ w1252]
                      tunnel: w1186 -> [_ w1251]
                      tunnel: [TRUE ("profile complete?") w1246] -> w1176
                      tunnel: w1184 -> [w1191 w1248]
                      tunnel: [w1200 w1245] -> w1183
                      tunnel: [FALSE w1243] -> w1182
                      tunnel: [w1202 w1243] -> w1181
                      tunnel: [0.0 ("u") w1249] -> w1180
                      tunnel: w1179 -> [w1193 w1241]
                      tunnel: w1178 -> [w1197 w1247]
                      tunnel: [w1196 w1244] -> w1177
                      tunnel: w1175 -> [w1195 w1242]
                      frame "Active", "Passive" {
                        # "Left Hand?"
                        n355 = Equal?(x=w1191, y=i16 1) -> (x = y?=w1192:bool)
                        n356 = Equal To 0?(x=w1193) -> (x = 0?=w1194:bool)
                        n357 = local read "StartSignal"() -> (w1205:bool)
                        n358 = And "first passive iteration?"(x=w1192, y=w1194) -> (x .and. y?=w1189:bool)
                        n359 = case shown="True" w1205 {
                          tunnel: w1191 -> [w1224 w1225]
                          tunnel: [FALSE TRUE] -> w1202
                          tunnel: [w1224 w1227] -> w1200
                          tunnel: w1198 -> [_ w1228]
                          tunnel: w1197 -> [w1222 w1226]
                          tunnel: [w1222 w1226] -> w1196
                          frame False {
                            # "Ongoing trial"
                          }
                          frame True {
                            # "User finished trial, switch to next subtask if this was 3rd trial"
                            n360 = Equal?(x=w1225, y=w1226) -> (x = y?=w1230:bool)
                            n361 = case shown="True" w1230 {
                              tunnel: w1228 -> [_ w1236]
                              tunnel: w1225 -> [w1232 _]
                              tunnel: [w1231 i16 1] -> w1227
                              frame False {
                                n362 = Increment(x=w1232) -> (x+1=w1231:i16)
                              }
                              frame True {
                                n363 = case shown="\"Passive\"" w1236 {
                                selector: w1236 -> [_ _ w1239]
                                tunnel: [ROM_States."Passive" ("ROM State") ROM_States."AutomaticPassive" ("ROM State") w1239] -> w1235
                                frame "Active" {
                                }
                                frame "Passive" {
                                }
                                frame "AutomaticPassive" {
                                }
                                }
                                n364 = local write "StartSignal"(FALSE ("StartSignal")) -> ()
                                n365 = local write "ROM State"(w1235) -> ()
                              }
                            }
                          }
                        }
                        n366 = case "Calculate ROM during passive motion" shown="\"Passive\"" w1198 {
                          tunnel: w1199 -> [_ w1211]
                          tunnel: w1195 -> [_ w1207]
                          tunnel: w1189 -> [_ w1206]
                          frame Default {
                          }
                          frame "Passive" {
                            n367 = case shown="True" w1206 {
                              tunnel: w1211 -> [w1220 w1221]
                              tunnel: [w1220 w1221] -> w1210
                              tunnel: [w1219 w1221] -> w1209
                              tunnel: [w1218 w1221] -> w1208
                              frame False {
                                n368 = local read "ROM max"() -> (w1219:dbl)
                                n369 = local read "ROM min"() -> (w1218:dbl)
                              }
                              frame True {
                                "ROM max" <- w1221
                                "ROM min" <- w1221
                              }
                            }
                            n370 = Max & Min(x=w1209, y=w1210) -> (max(x,y)=w1215:dbl, min(x,y)=w1216:dbl)
                            n371 = Max & Min(x=w1210, y=w1208) -> (max(x,y)=w1212:dbl, min(x,y)=w1213:dbl)
                            n372 = Select(t=w1215, s=w1207, f=w1216) -> (s? t:f=w1217:dbl)
                            n373 = Select(t=w1213, s=w1207, f=w1212) -> (s? t:f=w1214:dbl)
                            n374 = local write "ROM max"(w1217) -> ()
                            n375 = local write "ROM min"(w1214) -> ()
                          }
                        }
                      }
                      frame "AutomaticPassive" {
                        # "Generates a sinewave with the determined max range of motion"
                        n376 = Equal To 0?(x=w1241) -> (x = 0?=w1240:bool)
                        n377 = flat-sequence "Calculate and execute sinewave" {
                          tunnel: w1252 -> [w1271]
                          tunnel: w1251 -> [w1270]
                          tunnel: w1250 -> [w1269]
                          tunnel: [w1268] -> w1249
                          tunnel: [w1256] -> w1246
                          tunnel: w1242 -> [w1267]
                          tunnel: w1240 -> [w1253]
                          frame #0 {
                            w1264 = T42 {"output high"=1.4, "output low"=-1.4}  # Output range
                            n378 = feedback #5() -> (w1266:cluster{"time (s)":dbl, "setpoint":dbl}[])  [unwired: 1 in]
                            n379 = case shown="True" w1253 {
                              tunnel: [w1272 w1286] -> w1265
                              tunnel: w1266 -> [w1272 _]
                              tunnel: w1267 -> [_ w1275]
                              frame False {
                              }
                              frame True {
                                # "Sine wave amplitude"
                                # "2s movement \n(1s between flexion \n& extension)"
                                n380 = local read "ROM max"() -> (w1281:dbl)
                                n381 = local read "ROM min"() -> (w1277:dbl)
                                n382 = Subtract(x=w1281, y=w1277) -> (x-y=w1279:dbl)
                                n383 = Absolute Value(x=w1279) -> (abs(x)=w1280:dbl)
                                n384 = Divide(x=w1280, y=2.0) -> (x/y=w1273:dbl)
                                n385 = local read "Zero Position"() -> (w1283:dbl)
                                n386 = Negate(x=w1273) -> (-x=w1276:dbl)
                                n387 = Select(t=w1273, s=w1275, f=w1276) -> (s? t:f=w1274:dbl)
                                n388 = call "Sine_Trajectory.vi"("Amplitude"=w1274, "Offset"=w1283, "Frequency (Hz)"=1.0, "Duration (s)"=2.0, "Period (s)"=0.001) -> ("Profile"=w1286:cluster{"time (s)":dbl, "setpoint":dbl}[])  [unwired: 6 in]
                              }
                            }
                            n389 = feedback-in #5(w1265) -> ()
                            n390 = feedback #6() -> (w1254:bool)  [unwired: 1 in]
                            n391 = Or(x=w1253, y=w1254) -> (x .or. y?=w1255:bool)
                            n392 = call "sine_params.vi"() -> ("Gains"=w1263:T43, "Non-linear gain"=w1262:T44, "D-Part variable"=w1261:T46, "Velocity estimate dy/dt"=w1260:T47, "Anti reset windup"=w1259:bool, "I-Part error band"=w1258:dbl)  [unwired: 14 in]
                            n393 = call <vilib>:"PID Setpoint Profile.vi"("reinitialize? (F)"=w1255, "setpoint profile"=w1265) -> ("profile complete?"=w1256:bool, "setpoint"=w1257:dbl)  [unwired: 4 in, 2 out]
                            n394 = feedback-in #6(w1256) -> ()
                            n395 = call "ENPIDv2.vi"("Gains"=w1263, "Non-linear gain"=w1262, "D-Part variable"=w1261, "Velocity estimate dy/dt"=w1260, "Anti reset windup"=w1259, "I-Part error band"=w1258, "Output range"=w1264, "y"=w1269, "r"=w1257, "dy/dt"=w1270, "dt (s)"=w1271) -> ("u"=w1268:dbl)  [unwired: 7 in, 1 out]
                          }
                        }
                        n396 = case shown="True" w1246 {
                          tunnel: w1248 -> [w1289 w1290]
                          tunnel: w1247 -> [w1288 w1292]
                          tunnel: [w1289 w1293] -> w1245
                          tunnel: [w1288 w1292] -> w1244
                          tunnel: [FALSE w1291] -> w1243
                          frame False {
                          }
                          frame True {
                            n397 = Equal?(x=w1290, y=w1292) -> (x = y?=w1294:bool)
                            n398 = case "Finish up Task" shown="True" w1294 {
                              tunnel: [w1295 i16 0 ("Trial Nr")] -> w1293
                              tunnel: w1290 -> [w1296 _]
                              tunnel: [FALSE TRUE] -> w1291
                              frame False {
                                n399 = Increment(x=w1296) -> (x+1=w1295:i16)
                              }
                              frame True {
                                n400 = local write "StartSignal"(FALSE) -> ()
                              }
                            }
                          }
                        }
                      }
                    }
                  }
                  frame "Force" {
                    # "Increment TrialNr\nif cycles reached and not last trial"
                    # "Finish Trial after the\nset amount of cycles"
                    n401 = Multiply(x=w1302, y=i16 2) -> (x*y=w1303:i16)
                    n402 = Equal?(x=w1301, y=w1303) -> (x = y?=w1310:bool)
                    n403 = Equal?(x=w1312, y=3000) -> (x = y?=w1308:bool)
                    n404 = Not(x=w1310) -> (.not. x?=w1309:bool)
                    n405 = And(x=w1309, y=w1308) -> (x .and. y?=w1306:bool)
                    n406 = case "Trial Increment" shown="True" w1306 {
                      tunnel: w1301 -> [w1314 w1316]
                      tunnel: [w1314 w1315] -> w1307
                      frame False {
                      }
                      frame True {
                        n407 = Increment(x=w1316) -> (x+1=w1315:i16)
                      }
                    }
                  }
                  frame "PreciseReaching" {
                    # "Trial Finished"
                    # "Increment Trial Count\nif cycles reached and not last trial"
                    # "Trial Nr"
                    # "Finish Trial once we get another\nstart signal"
                    n408 = Multiply(x=i16 2, y=w1319) -> (x*y=w1321:i16)
                    n409 = local read "StartSignal"() -> (w1318:bool)
                    n410 = Equal? "Max Trials Reached"(x=w1317, y=w1321) -> (x = y?=w1325:bool)
                    n411 = Not(x=w1325) -> (.not. x?=w1324:bool)
                    n412 = And(x=w1324, y=w1318) -> (x .and. y?=w1322:bool)
                    n413 = case "Trial Increment" shown="True" w1322 {
                      tunnel: w1317 -> [w1328 w1330]
                      tunnel: [w1328 w1329] -> w1323
                      frame False {
                      }
                      frame True {
                        n414 = Increment(x=w1330) -> (x+1=w1329:i16)
                      }
                    }
                  }
                  frame "Motor", Default {
                    # "Trial Finished"
                    # "Increment Trial Count\nif cycles reached and not last trial"
                    # "Trial Nr"
                    # "Finish Trial after 4 seconds"
                    n415 = Greater Or Equal?(x=w1334, y=4000) -> (x >= y?=w1332:bool)
                    n416 = Multiply(x=i16 2, y=w1335) -> (x*y=w1337:i16)
                    n417 = Equal? "Max Trials Reached"(x=w1331, y=w1337) -> (x = y?=w1341:bool)
                    n418 = Not(x=w1341) -> (.not. x?=w1340:bool)
                    n419 = And(x=w1340, y=w1332) -> (x .and. y?=w1338:bool)
                    n420 = case "Trial Increment" shown="True" w1338 {
                      tunnel: w1331 -> [w1344 w1346]
                      tunnel: [w1344 w1345] -> w1339
                      frame False {
                      }
                      frame True {
                        n421 = Increment(x=w1346) -> (x+1=w1345:i16)
                      }
                    }
                  }
                  frame "Sensorimotor" {
                    w1356 = 0.0008377580409572782  # (2*pi*4) / 30'000
                    w1355 = 0.0004188790204786391  # (2*pi*2) / 30'000
                    w1354 = 0.00020943951023931956  # (2*pi*1) / 30'000
                    # "Increment Trial when finished\nand not last trial"
                    n422 = Equal To 0?(x=w1373) -> (x = 0?=w1372:bool)
                    n423 = call "Tick Count3"() -> ("Tick Count(mSec)"=w1370:u32)
                    n424 = Less Or Equal? "InSlowPhase"(x=w1347, y=w1384) -> (x <= y?=w1386:bool)
                    n425 = feedback #7() -> (w1371:u32)  [unwired: 1 in]
                    n426 = Select(t=w1370, s=w1372, f=w1371) -> (s? t:f=w1369:u32)
                    n427 = feedback-in #7(w1369) -> ()
                    n428 = Subtract "ms since start"(x=w1370, y=w1369) -> (x-y=w1364:u32)
                    n429 = Select(t=u32 1, s=w1386, f=u32 3) -> (s? t:f=w1365:u32)
                    n430 = Multiply "speedmul * t"(x=w1365, y=w1364) -> (x*y=w1358:u32)
                    n431 = Greater Or Equal? "IsComplete?"(x=w1364, y=u32 30000) -> (x >= y?=w1363:bool)
                    n432 = To Double Precision Float(number=w1358) -> (double precision float=w1357:dbl)
                    n433 = Multiply(x=w1357, y=w1354) -> (x*y=w1361:dbl)
                    n434 = Multiply(x=w1357, y=w1355) -> (x*y=w1360:dbl)
                    n435 = Multiply(x=w1357, y=w1356) -> (x*y=w1359:dbl)
                    n436 = Sine(x=w1360) -> (sin(x)=w1377:dbl)
                    n437 = Sine(x=w1359) -> (sin(x)=w1375:dbl)
                    n438 = Sine(x=w1361) -> (sin(x)=w1378:dbl)
                    n439 = local read "Starting position"() -> (w1374:dbl)
                    n440 = Add(x=w1378, y=w1377) -> (x+y=w1376:dbl)
                    n441 = Multiply(x=i16 2 ("y"), y=w1384) -> (x*y=w1385:i16)
                    n442 = Add(x=w1376, y=w1375) -> (x+y=w1353:dbl)
                    n443 = Select(t=15.0 ("x"), s=w1348, f=-15.0 ("x")) -> (s? t:f=w1349:dbl)
                    n444 = Multiply(x=w1349, y=w1353) -> (x*y=w1352:dbl)
                    n445 = Equal? "Max Trials Reached"(x=w1347, y=w1385) -> (x = y?=w1382:bool)
                    n446 = Add(x=w1352, y=w1374) -> (x+y=w1362:dbl)
                    n447 = local write "Target Position [deg]"(w1362) -> ()
                    n448 = Not(x=w1382) -> (.not. x?=w1387:bool)
                    n449 = And(x=w1387, y=w1363) -> (x .and. y?=w1381:bool)
                    n450 = Increment(x=w1347) -> (x+1=w1380:i16)
                    n451 = Select(t=w1380, s=w1381, f=w1347) -> (s? t:f=w1379:i16)
                  }
                  frame "PositionMatching" {
                    w1404 = T42 {"output high"=5.0, "output low"=-5.0}  # Output range
                    # "Read actual Target Element from Array\n(Array starts from 0, Trial from 1)"
                    n452 = Equal To 0? "First Iteration"(x=w1410) -> (x = 0?=w1409:bool)
                    n453 = local read "Target Array"() -> (w1411:dbl[])
                    n454 = Decrement(x=w1418) -> (x-1=w1395:i16)
                    n455 = To Long Integer(number=w1395) -> (32bit integer=w1394:i32)
                    n456 = case "Check if first Iteration of Trial" shown="False" w1409 {
                      tunnel: [w1421 w1422] -> w1406
                      frame False {
                        n457 = local read "MovingToTarget"() -> (w1421:bool)
                      }
                      frame True {
                        w1422 = TRUE ("FirstRound")
                        "MovingToTarget" <- w1422
                      }
                    }
                    n458 = Index Array(array=w1411, index=w1394) -> (element=w1419:dbl)
                    n459 = case "Deactivates StartSignal\nuntil moving is completed" shown="True" w1406 {
                      tunnel: [w1423 FALSE ("Boolean")] -> w1405
                      frame False {
                        # "StartSignal acts \nas finish signal"
                        n460 = local read "StartSignal"() -> (w1423:bool)
                      }
                      frame True {
                      }
                    }
                    n461 = feedback #8() -> (w1417:cluster{"time (s)":dbl, "setpoint":dbl}[])  [unwired: 1 in]
                    n462 = feedback #9(TRUE ("profile complete?")) -> (w1414:bool)
                    n463 = Or(x=w1409, y=w1414) -> (x .or. y?=w1413:bool)
                    n464 = case shown="True" w1413 {
                      tunnel: [w1427 w1429] -> w1416
                      tunnel: w1417 -> [w1427 _]
                      tunnel: w1390 -> [_ w1430]
                      tunnel: w1419 -> [_ w1428]
                      frame False {
                      }
                      frame True {
                        n465 = local write "Target Position [deg]"(w1428) -> ()
                        n466 = call "motion_create_minimum_jerk.vi"("Initial Position"=w1430, "Final Position"=w1428, "Initial Time [s]"=0.0, "Final Time [s]"=3.0, "Delta Time [s]"=0.01) -> ("Profile"=w1429:cluster{"time (s)":dbl, "setpoint":dbl}[])  [unwired: 10 in]
                      }
                    }
                    n467 = feedback-in #8(w1416) -> ()
                    n468 = call <vilib>:"PID Setpoint Profile.vi"("reinitialize? (F)"=w1413, "setpoint profile"=w1416) -> ("profile complete?"=w1391:bool, "setpoint"=w1396:dbl)  [unwired: 4 in, 2 out]
                    n469 = feedback-in #9(w1391) -> ()
                    n470 = call "min_jerk_params.vi"() -> ("Gains"=w1403:T43, "Non-linear gain"=w1402:T44, "D-Part variable"=w1401:T46, "Velocity estimate dy/dt"=w1400:T47, "Anti reset windup"=w1399:bool, "I-Part error band"=w1398:dbl)  [unwired: 14 in]
                    n471 = call "ENPIDv2.vi"("Gains"=w1403, "Non-linear gain"=w1402, "D-Part variable"=w1401, "Velocity estimate dy/dt"=w1400, "Anti reset windup"=w1399, "I-Part error band"=w1398, "Output range"=w1404, "y"=w1390, "r"=w1396, "dy/dt"=w1393, "dt (s)"=w1397) -> ("u"=w1392:dbl)  [unwired: 7 in, 1 out]
                    n472 = And(x=w1406, y=w1391) -> (x .and. y?=w1412:bool)
                    n473 = case "Finish Trial" shown="True" w1405 {
                      tunnel: w1418 -> [w1434 w1437]
                      tunnel: [w1434 w1436] -> w1408
                      frame False {
                      }
                      frame True {
                        n474 = Increment(x=w1437) -> (x+1=w1436:i16)
                        n475 = local write "Target state?"(FALSE ("TargetState")) -> ()
                      }
                    }
                    n476 = case "Start Probe" shown="True" w1412 {
                      frame False {
                      }
                      frame True {
                        n477 = local write "Target state?"(TRUE ("TargetState")) -> ()
                        n478 = local write "MovingToTarget"(FALSE ("FirstRound")) -> ()
                      }
                    }
                    n479 = Greater?(x=w1408, y=w1407) -> (0:w1420:bool)
                  }
                }
                n480 = disable-structure shown="Enabled" {
                  disable-tunnel: [w1439 0.0 ("Current")] -> w1159
                  disable-tunnel: w1153 -> [w1438 _]
                  frame Enabled {
                    # "Position"
                    # "Disable this Subdiagram to deactivate gravity compensation"
                    n481 = call "GravityCompensation.vi"("Position [deg]"=w1438) -> ("Current"=w1439:dbl)
                  }
                  frame Disabled {
                  }
                }
                n482 = And(x=w1164, y=w1148) -> (x .and. y?=w1149:bool)
                n483 = case shown="False" w1149 {
                  tunnel: w1148 -> [w1167 _]
                  tunnel: [w1168 Main_States."Resetting" ("Task states")] -> w1147
                  frame False {
                    # "Assessment Running"
                    n484 = case shown="True" w1167 {
                      tunnel: [Main_States."Show target" ("Task states") Main_States."Start" ("Task states")] -> w1168
                      frame False {
                        # "Trial Running"
                      }
                      frame True {
                        # "Trial Finished"
                        n485 = local write "Target state?"(FALSE ("Target state?")) -> ()
                        n486 = local write "SkipSignal"(FALSE ("SkipSignal")) -> ()
                      }
                    }
                  }
                  frame True {
                    # "Assessment Finished"
                    n487 = local write "AssessmentFinished"(TRUE ("AssessmentFinished")) -> ()
                  }
                }
                n488 = Increment(x=w1152) -> (x+1=w1150:i32)
                n489 = Select(t=w1159, s=w1161, f=w1160) -> (s? t:f=w1162:dbl)
              }
              frame "Resetting" {
                w1442 = FALSE ("Target state?")
                # "Clear Patient Data and reset other state"
                n490 = local write "FrontendStartedSignal"(w1442) -> ()
                n491 = local write "SelectedHand"(Hand."None" ("SelectedHand")) -> ()
                n492 = local write "Target state?"(w1442) -> ()
                n493 = local write "SkipSignal"(w1442) -> ()
                n494 = local write "ROM State"(ROM_States."Active" ("ROM State")) -> ()
                n495 = local write "LeftHand"(w1442) -> ()
              }
              frame "WaitingForRestart" {
                # "Current Task State"
                n496 = local read "RestartSignal"() -> (w1453:bool)
                n497 = local read "LogFileOpen"() -> (w1455:bool)
                n498 = Not(x=w1455) -> (.not. x?=w1454:bool)
                n499 = And(x=w1453, y=w1454) -> (x .and. y?=w1452:bool)
                n500 = case shown="True" w1452 {
                  tunnel: w1451 -> [w1461 _]
                  tunnel: [w1461 Main_States."Hand choice" ("Task states")] -> w1450
                  frame False {
                    # "Waiting for restart"
                  }
                  frame True {
                    # "Restart State Machine"
                    n501 = flat-sequence {
                      tunnel: FALSE ("Target state?") -> [w1465]
                      tunnel: [w1465] -> w1462
                      frame #0 {
                        n502 = local write "AssessmentFinished"(w1465) -> ()
                      }
                    }
                    n503 = local write "RestartSignal"(w1462) -> ()
                  }
                }
              }
            }
          }
          frame #3 {
            w1473 = -10.0  # [V]
            w1472 = 10.0  # [V]
            # "Safety"
            # "Task State"
            # "Phase Trial Count"
            # "Assessment Mode"
            # "Trial Nr"
            # "Position"
            # "Loop count"
            # "Motor Current Setpoint"
            # "Send Motor Command"
            n504 = call "TF_MotorCurrentOutput.vi"("Motor Current Setpoint [A]"=w1487) -> ("Motor Current Setpoint [V]"=w1486:dbl)
            n505 = local read "RestartSignal"() -> (w1476:bool)
            n506 = Not Equal?(x=Main_States."WaitingForRestart" ("Task states"), y=w1478) -> (x != y?=w1477:bool)
            n507 = And(x=w1477, y=w1476) -> (x .and. y?=w1475:bool)
            n508 = Absolute Value(x=w1489) -> (abs(x)=w1470:dbl)
            n509 = local read "StopSignal"() -> (w1483:bool)
            n510 = case "Initiate restart procedure" shown="True" w1475 {
              tunnel: w1478 -> [w1493 _]
              tunnel: [w1493 Main_States."Resetting" ("t")] -> w1474
              frame False {
              }
              frame True {
              }
            }
            "Task State" <- w1474
            n511 = In Range and Coerce(upper limit=w1472, x=w1486, lower limit=w1473) -> (coerced(x)=w1471:dbl)  [unwired: 1 out]
            n512 = Less Or Equal?(x=w1470, y=w1467) -> (x <= y?=w1469:bool)
            n513 = Or(x="stop", y=w1483) -> (x .or. y?=w1485:bool)
            "StopRequested" <- w1485
            n514 = Select(t=w1471, s=w1469, f=0.0) -> (s? t:f=w1466:dbl)
            n515 = Build Array(w1466) -> (w1492:dbl[])
            n516 = call <vilib>:"Write.vi"("Values"=w1492, "AO Ref In"=w1491) -> ("AO Ref Out"=w1490:T24)  [unwired: 7 in, 1 out]
            "Current Setpoint [A]" <- w1487
            "Trial Nr" <- w1482
          }
        }
        n517 = node-c288() -> ()  [unwired: 1 in, 1 out]
      }
      n518 = node-c288(w259) -> ()  [unwired: 1 out]
      n519 = node-c288(w286) -> ()  [unwired: 1 out]
      n520 = Build Array(0.0) -> (w247:dbl[])
      n521 = call <vilib>:"Write.vi"("Values"=w247, "AO Ref In"=w249) -> ("AO Ref Out"=w248:T24)  [unwired: 7 in, 1 out]
      "Velocity_calib_value" <- w255
      "Force_calib_value" <- w245
    }
    frame #5 {
      # "Close UDP Socket"
      # "Close TCP Listener"
      # "Reset"
      # "Force Sensor"
      # "Tachometer"
      # "Motor Current Monitor"
      # "Motor Current Setpoint"
      # "Encoder"
      # "Close everything"
      n522 = Release Notifier(notifier=w1507) -> ()  [unwired: 2 in, 3 out]
      n523 = TCP Close Connection(connection ID=w1510) -> (error out=w1508:errorcluster)  [unwired: 2 in, 1 out]
      n524 = UDP Close(connection ID=w1511) -> (error out=w1509:errorcluster)  [unwired: 1 in, 1 out]
      n525 = RT FIFO Delete(0:w1506) -> ()  [unwired: 2 in, 1 out]
      n526 = call <vilib>:"Close.vi"("AO Ref In"=w1515) -> ()  [unwired: 10 in, 1 out]
      n527 = call <vilib>:"Close.vi"("AO Ref In"=w1505) -> ()  [unwired: 10 in, 1 out]
      n528 = call <vilib>:"Stop.vi"("Encoder Ref In"=w1516) -> ("Encoder Ref Out"=w1517:T32)  [unwired: 9 in, 1 out]
      n529 = call <vilib>:"Close.vi"("AI Ref In"=w1512) -> ()  [unwired: 10 in, 1 out]
      n530 = call <vilib>:"Close.vi"("AI Ref In"=w1514) -> ()  [unwired: 10 in, 1 out]
      n531 = call <vilib>:"Close.vi"("AI Ref In"=w1513) -> ()  [unwired: 10 in, 1 out]
      n532 = local write "UDP Error"(w1509) -> ()
      n533 = local write "TCP Error"(w1508) -> ()
      n534 = call <vilib>:"Close.vi"("Encoder Ref In"=w1517) -> ()  [unwired: 10 in, 1 out]
    }
  }
